vi "Parse Uplink.vi"(8 "error in (no error)":errorcluster, 10 "Uplink":u8[][](array[numeric]) format="%02x") -> (0 "error out":errorcluster, 1 "Data":string, 2 "Response Code":string, 3 "Response Token":string, 4 "tChecksum Valid":bool, 5 "CP_DATA":u8[](array[numeric]), 6 "bChecksum Valid":bool)   [LabVIEW 2020]
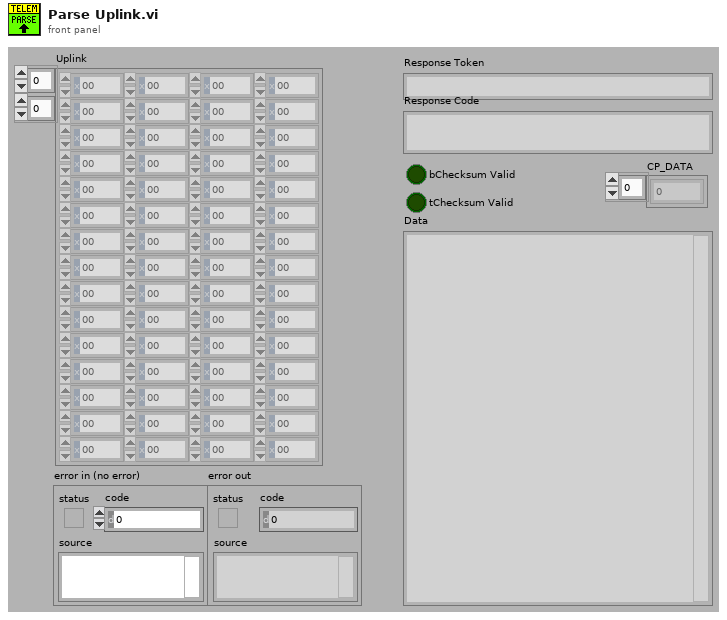
[diagram p1: front panel]
types:
  T1 = cluster{"FirstBlockFlag":u8, "respToken":u8, "cmdToken":u16, "cmdData":u8[], "b1ChkSum":u8, "tChkSum":u8, "tChkSumCalc":u8, "b1ChkSumCalc":u8}
  T2 = cluster{"Boolean array[0]":bool, "Boolean array[1]":bool, "Boolean array[2]":bool, "Boolean array[3]":bool, "Boolean array[4]":bool, "Boolean array[5]":bool, "Boolean array[6]":bool, "Boolean array[7]":bool}
  T3 = cluster{"Boolean array[0]":bool, "Boolean array[1]":bool, "Boolean array[2]":bool, "Boolean array[3]":bool, "Boolean array[4]":bool, "Boolean array[5]":bool, "Boolean array[6]":bool, "Boolean array[7]":bool, "Boolean array[8]":bool, "Boolean array[9]":bool, "Boolean array[10]":bool, "Boolean array[11]":bool, "Boolean array[12]":bool, "Boolean array[13]":bool, "Boolean array[14]":bool, "Boolean array[15]":bool}
  T4 = cluster{"DATA[0]":u8, "DATA[1]":u8, "DATA[2]":u8, "DATA[3]":u8, "DATA[4]":u8, "DATA[5]":u8, "DATA[6]":u8, "DATA[7]":u8}
  T5 = cluster{"[0]":string, "[1]":string, "[2]":string, "[3]":string, "[4]":string, "[5]":string, "[6]":string, "[7]":string, "[8]":string, "[9]":string}
  T6 = cluster{"DATA[0]":u8, "DATA[1]":u8, "DATA[2]":u8, "DATA[3]":u8, "DATA[4]":u8, "DATA[5]":u8, "DATA[6]":u8, "DATA[7]":u8, "DATA[8]":u8, "DATA[9]":u8, "DATA[10]":u8, "DATA[11]":u8, "DATA[12]":u8, "DATA[13]":u8, "DATA[14]":u8, "DATA[15]":u8}
  T7 = cluster{"[0]":u8, "[1]":u8, "[2]":u8, "[3]":u8, "[4]":u8, "[5]":u8, "[6]":u8, "[7]":u8, "[8]":u8, "[9]":u8, "[10]":u8, "[11]":u8, "[12]":u8, "[13]":u8, "[14]":u8, "[15]":u8, "[16]":u8, "[17]":u8, "[18]":u8, "[19]":u8, "[20]":u8, "[21]":u8, "[22]":u8, "[23]":u8, "[24]":u8, "[25]":u8, "[26]":u8, "[27]":u8, "[28]":u8, "[29]":u8, "[30]":u8, "[31]":u8, "[32]":u8, "[33]":u8, "[34]":u8, "[35]":u8, "[36]":u8, "[37]":u8, "[38]":u8, "[39]":u8, "[40]":u8, "[41]":u8, "[42]":u8, "[43]":u8, "[44]":u8, "[45]":u8, "[46]":u8, "[47]":u8, "[48]":u8, "[49]":u8, "[50]":u8, "[51]":u8, "[52]":u8, "[53]":u8}
  T8 = cluster{"DATA[0]":u8, "DATA[1]":u8, "DATA[2]":u8, "DATA[3]":u8, "DATA[4]":u8, "DATA[5]":u8, "DATA[6]":u8, "DATA[7]":u8, "DATA[8]":u8, "DATA[9]":u8, "DATA[10]":u8, "DATA[11]":u8, "DATA[12]":u8, "DATA[13]":u8, "DATA[14]":u8, "DATA[15]":u8, "DATA[16]":u8, "DATA[17]":u8, "DATA[18]":u8, "DATA[19]":u8, "DATA[20]":u8, "DATA[21]":u8, "DATA[22]":u8, "DATA[23]":u8, "DATA[24]":u8, "DATA[25]":u8, "DATA[26]":u8, "DATA[27]":u8, "DATA[28]":u8, "DATA[29]":u8, "DATA[30]":u8, "DATA[31]":u8, "DATA[32]":u8, "DATA[33]":u8, "DATA[34]":u8, "DATA[35]":u8, "DATA[36]":u8, "DATA[37]":u8, "DATA[38]":u8, "DATA[39]":u8, "DATA[40]":u8, "DATA[41]":u8, "DATA[42]":u8, "DATA[43]":u8, "DATA[44]":u8, "DATA[45]":u8, "DATA[46]":u8}
  T9 = cluster{"DATA[0]":u8, "DATA[1]":u8, "DATA[2]":u8, "DATA[3]":u8, "DATA[4]":u8, "DATA[5]":u8, "DATA[6]":u8, "DATA[7]":u8, "DATA[8]":u8, "DATA[9]":u8, "DATA[10]":u8, "DATA[11]":u8, "DATA[12]":u8, "DATA[13]":u8, "DATA[14]":u8, "DATA[15]":u8, "DATA[16]":u8, "DATA[17]":u8, "DATA[18]":u8, "DATA[19]":u8, "DATA[20]":u8, "DATA[21]":u8, "DATA[22]":u8, "DATA[23]":u8}
  T10 = cluster{"Boolean array[0]":bool, "Boolean array[1]":bool, "Boolean array[2]":bool, "Boolean array[3]":bool, "Boolean array[4]":bool, "Boolean array[5]":bool, "Boolean array[6]":bool, "Boolean array[7]":bool, "Boolean array[8]":bool}
  T11 = cluster{"[0]":u8, "[1]":u8, "[2]":u8, "[3]":u8, "[4]":u8, "[5]":u8, "[6]":u8, "[7]":u8, "[8]":u8, "[9]":u8}
  T12 = cluster{"DATA[0]":u8, "DATA[1]":u8, "DATA[2]":u8, "DATA[3]":u8, "DATA[4]":u8, "DATA[5]":u8, "DATA[6]":u8, "DATA[7]":u8, "DATA[8]":u8}
  T13 = cluster{"[0]":u8, "[1]":u8, "[2]":u8, "[3]":u8, "[4]":u8, "[5]":u8, "[6]":u8, "[7]":u8, "[8]":u8, "[9]":u8, "[10]":u8, "[11]":u8, "[12]":u8, "[13]":u8, "[14]":u8, "[15]":u8, "[16]":u8, "[17]":u8, "[18]":u8, "[19]":u8, "[20]":u8, "[21]":u8, "[22]":u8, "[23]":u8, "[24]":u8, "[25]":u8, "[26]":u8, "[27]":u8, "[28]":u8, "[29]":u8, "[30]":u8, "[31]":u8, "[32]":u8, "[33]":u8, "[34]":u8, "[35]":u8, "[36]":u8, "[37]":u8}
  T14 = cluster{"[0]":u8, "[1]":u8, "[2]":u8, "[3]":u8, "[4]":u8, "[5]":u8}
  T15 = cluster{"DATA[0]":u8, "DATA[1]":u8, "DATA[2]":u8, "DATA[3]":u8, "DATA[4]":u8, "DATA[5]":u8}
  T16 = cluster{"DATA[0]":u8, "DATA[1]":u8, "DATA[2]":u8, "DATA[3]":u8, "DATA[4]":u8, "DATA[5]":u8, "DATA[6]":u8, "DATA[7]":u8, "DATA[8]":u8, "DATA[9]":u8, "DATA[10]":u8, "DATA[11]":u8, "DATA[12]":u8, "DATA[13]":u8, "DATA[14]":u8, "DATA[15]":u8, "DATA[16]":u8}
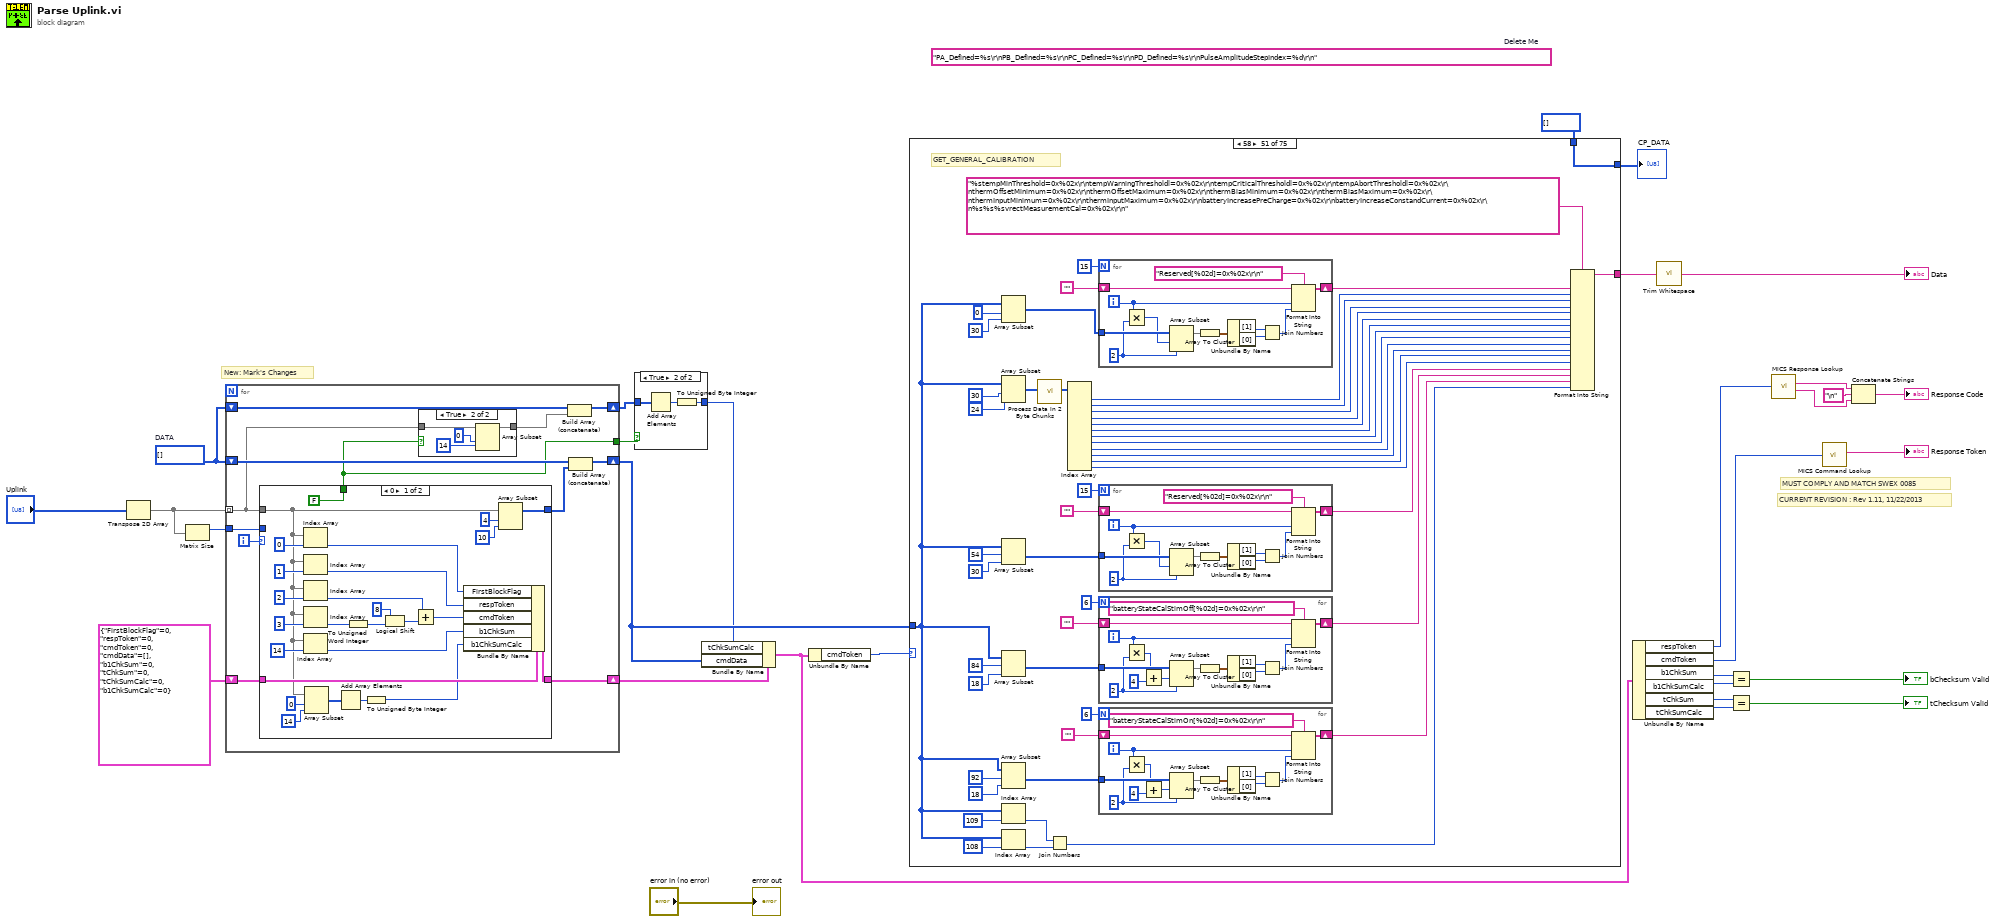
[diagram p0: block diagram]
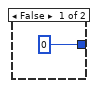
[diagram p2: hidden frame]
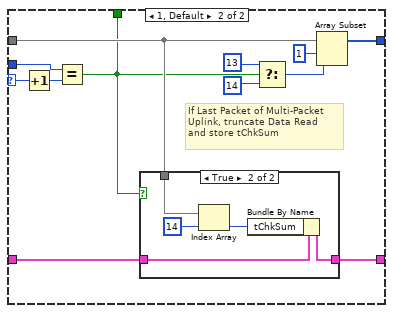
[diagram p4: hidden frame]
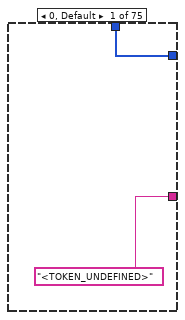
[diagram p6: hidden frame]
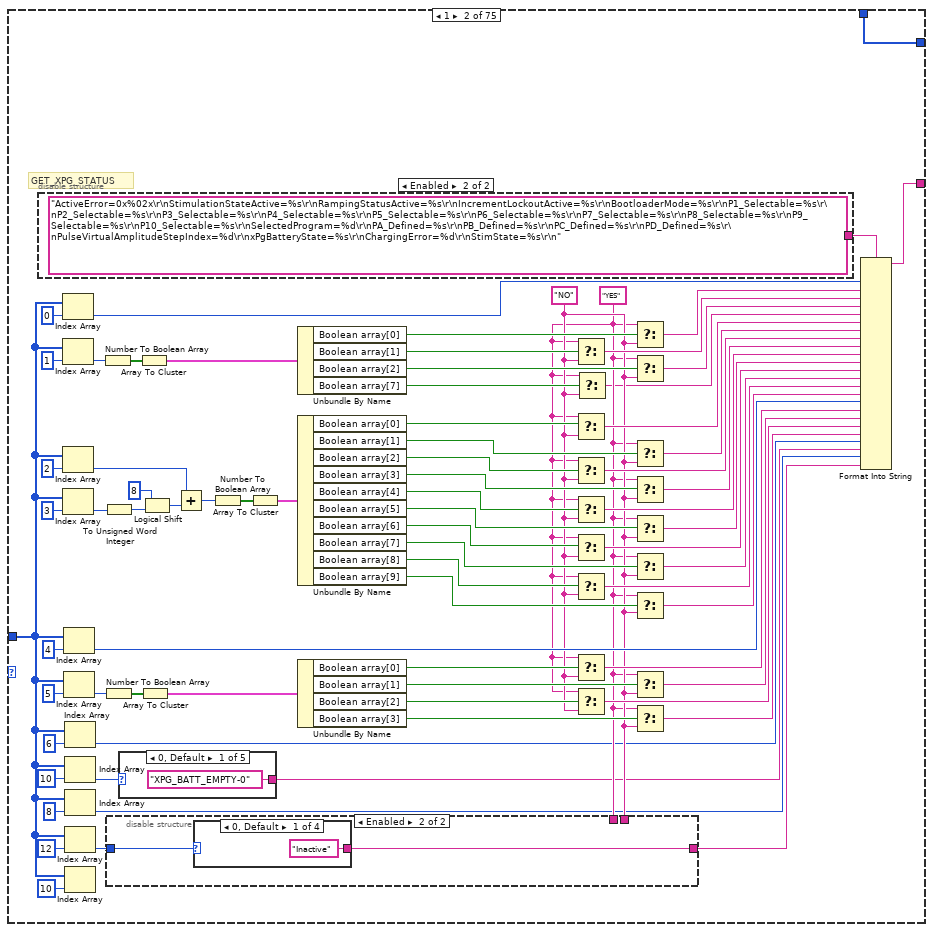
[diagram p7: hidden frame]
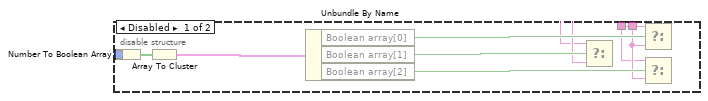
[diagram p8: hidden frame]
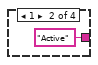
[diagram p9: hidden frame]
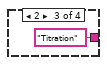
[diagram p10: hidden frame]
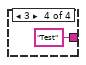
[diagram p11: hidden frame]
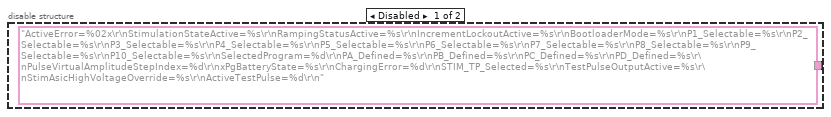
[diagram p12: hidden frame]
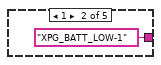
[diagram p13: hidden frame]
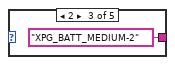
[diagram p14: hidden frame]
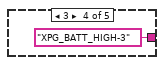
[diagram p15: hidden frame]
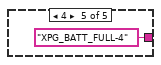
[diagram p16: hidden frame]
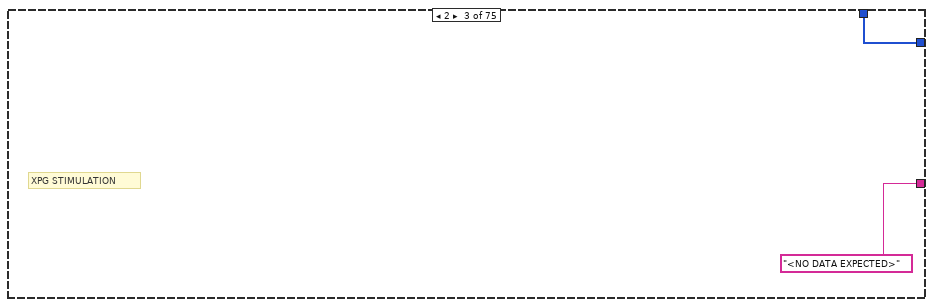
[diagram p17: hidden frame]
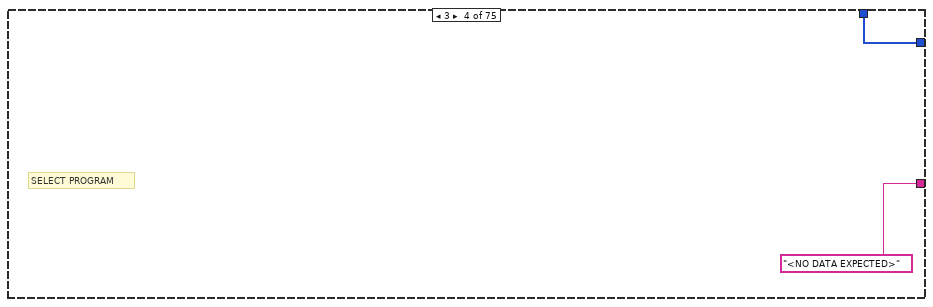
[diagram p18: hidden frame]
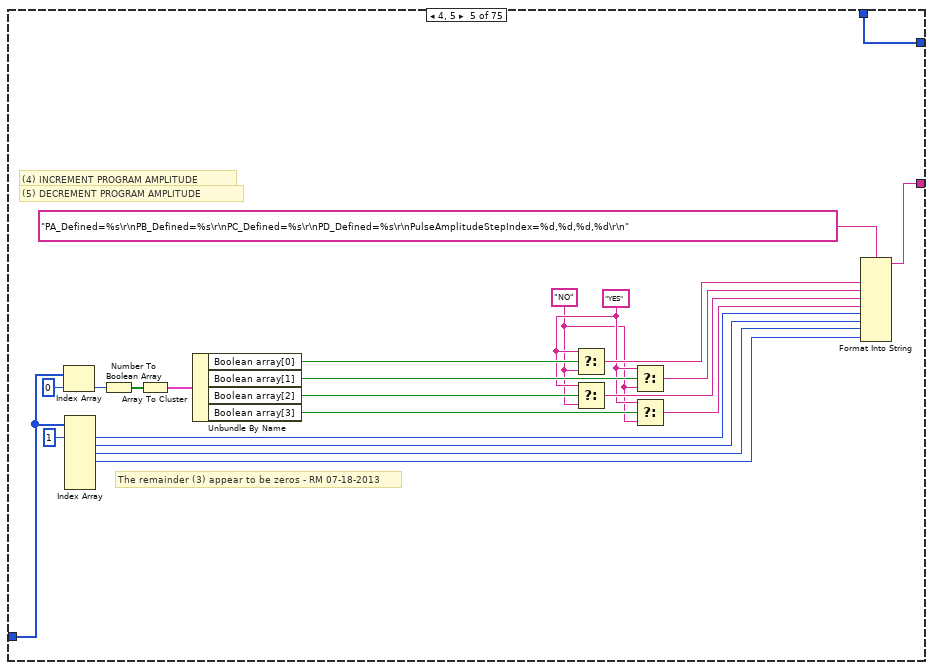
[diagram p19: hidden frame]
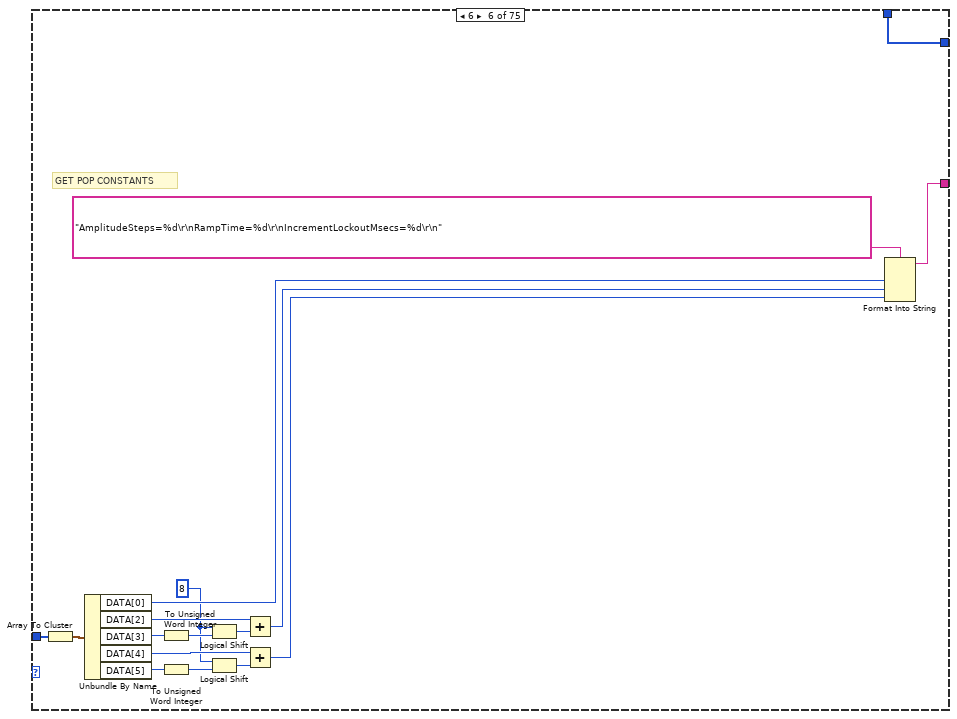
[diagram p20: hidden frame]
diagram:
  w14 = u8[] []  # DATA
  (unwired) "PA_Defined=%s\r\nPB_Defined=%s\r\nPC_Defined=%s\r\nPD_Defined=%s\r\nPulseAmplitudeStepIndex=%d\r\n"  # Delete Me
  # "CURRENT REVISION : Rev 1.11, 11/22/2013"
  # "MUST COMPLY AND MATCH SWEX 0085"
  # "New: Mark's Changes"
  n1 = Transpose 2D Array(2D array="Uplink") -> (transposed array=w13:u8[][])
  n2 = Matrix Size(0:w13) -> (1:w11:i32)  [unwired: 1 out]
  n3 = for {
    tunnel: w13 -> [w33] mode=indexing
    shift-right: [w37] -> w30
    shift-left: w14 -> [w38]
    shift-right: [w40] -> w12
    shift-left: T1 {"FirstBlockFlag"=0, "respToken"=0, "cmdToken"=0, "cmdData"=[], "b1ChkSum"=0, "tChkSum"=0, "tChkSumCalc"=0, "b1ChkSumCalc"=0} -> [w41]
    tunnel: w11 -> [w39]
    shift-right: [w34] -> w15
    shift-left: w14 -> [w35]
    tunnel: [w31] -> w16
    i -> [w42]
    n4 = case shown="0" w42 {
      selector: w42 -> [_ w85]
      tunnel: w33 -> [w51 w75]
      tunnel: [w71 w81] -> w36
      tunnel: w41 -> [w65 w76]
      tunnel: [w64 w77] -> w40
      tunnel: w39 -> [_ w83]
      tunnel: [FALSE w74] -> w31
      frame 0 {
        n5 = Index Array(array=w51, index=0) -> (element=w63:u8)
        n6 = Index Array(array=w51, index=1) -> (element=w60:u8)
        n7 = Index Array(array=w51, index=2) -> (element=w55:u8)
        n8 = Index Array(array=w51, index=3) -> (element=w59:u8)
        n9 = Index Array(array=w51, index=14) -> (element=w62:u8)
        n10 = Array Subset(array=w51, index=0, length=14) -> (w48:u8[])
        n11 = Add Array Elements(numeric array=w48) -> (sum=w50:u8)
        n12 = To Unsigned Word Integer(number=w59) -> (unsigned 16bit integer=w61:u16)
        n13 = To Unsigned Byte Integer(number=w50) -> (unsigned 8bit integer=w49:u8)
        n14 = Logical Shift(y=i8 8, x=w61) -> (x << y=w57:u16)
        n15 = Add(x=w55, y=w57) -> (x+y=w56:u16)
        n16 = Bundle By Name(cluster=w65, "FirstBlockFlag"=w63, "respToken"=w60, "cmdToken"=w56, "b1ChkSum"=w62, "b1ChkSumCalc"=w49) -> (w64:T1)
        n17 = Array Subset(array=w51, index=4, length=10) -> (w71:u8[])
      }
      frame 1, Default {
        # "If Last Packet of Multi-Packet\nUplink, truncate Data Read\nand store tChkSum"
        n18 = Increment(x=w85) -> (x+1=w84:i32)
        n19 = Equal?(x=w83, y=w84) -> (x = y?=w74:bool)
        n20 = case shown="True" w74 {
          tunnel: [w86 w90] -> w77
          tunnel: w76 -> [w86 w91]
          tunnel: w75 -> [_ w88]
          frame False {
          }
          frame True {
            n21 = Index Array(array=w88, index=14) -> (element=w89:u8)
            n22 = Bundle By Name(cluster=w91, "tChkSum"=w89) -> (w90:T1)
          }
        }
        n23 = Select(t=13 ("length"), s=w74, f=14 ("length")) -> (s? t:f=w80:i32)
        n24 = Array Subset(array=w75, index=1, length=w80) -> (w81:u8[])
      }
    }
    n25 = case shown="True" w31 {
      tunnel: w33 -> [w43 w46]
      tunnel: [w43 w45] -> w32
      frame False {
      }
      frame True {
        n26 = Array Subset(array=w46, index=0, length=14) -> (w45:u8[])
      }
    }
    n27 = Build Array (concatenate)(w35, w32) -> (w34:u8[])
    n28 = Build Array (concatenate)(w38, w36) -> (w37:u8[])
  }
  n29 = case shown="True" w16 {
    tunnel: w15 -> [_ w93]
    tunnel: [u16 0 ("CRC16r") w94] -> w17
    frame False {
    }
    frame True {
      n30 = Add Array Elements(numeric array=w93) -> (sum=w95:u8)
      n31 = To Unsigned Byte Integer(number=w95) -> (unsigned 8bit integer=w94:u8)
    }
  }
  n32 = Bundle By Name(cluster=w12, "tChkSumCalc"=w17, "cmdData"=w30) -> (w21:T1)
  n33 = Unbundle By Name(w21) -> ("cmdToken"=w18:u16)
  n34 = case shown="58" w18 {
    tunnel: w30 -> [_ w108 _ _ w209 w228 w238 w321 w368 w374 w380 w397 _ w418 w424 w430 _ w438 w444 _ w461 w488 _ _ w499 _ w638 _ w665 _ w817 _ w828 _ w888 _ w937 _ w971 _ _ w1002 w1037 w1060 w1081 _ w1091 _ w1103 w1109 w1131 _ w1219 _ w1269 _ w1276 _ w1338 _ w1396 _ w1403 _ _ _ w1424 _ _ _ _ w1447 _ w1505 _]
    tunnel: ["<TOKEN_UNDEFINED>" w170 "<NO DATA EXPECTED>" "<NO DATA EXPECTED>" w219 w235 w297 w354 w369 w375 w381 w411 "<NO DATA EXPECTED>" w419 w425 w431 "<NO DATA EXPECTED>" w439 w445 "<NO DATA EXPECTED>" w462 w475 "<NO DATA EXPECTED>" "<NO DATA EXPECTED>" w538 "<NO DATA EXPECTED>" w641 "<NO DATA EXPECTED>" w730 "<NO DATA EXPECTED>" w821 "<NO DATA EXPECTED>" w833 "<NO DATA EXPECTED>" w893 "<NO DATA EXPECTED>" w940 "<NO DATA EXPECTED>" w973 "<NO DATA EXPECTED>" "<NO DATA EXPECTED>" ("format string") w1003 w1039 w1062 w1083 "<NO DATA EXPECTED>" w1095 "<NO DATA EXPECTED>" w1105 w1113 w1162 "<NO DATA EXPECTED>" w1220 "<NO DATA EXPECTED>" w1270 "<NO DATA EXPECTED>" w1284 "<NO DATA EXPECTED>" w1345 "<NO DATA EXPECTED>" w1397 "<NO DATA EXPECTED>" w1411 _ _ "<NO DATA EXPECTED>" w1432 "<NO DATA EXPECTED>" _ _ _ w1448 "<NO DATA EXPECTED>" w1507 "<TOKEN_UNDEFINED (0x7FAA)>"] -> w29
    tunnel: [w96 w98 w193 w195 w197 w220 w237 w307 w365 w371 w377 w383 w413 w415 w421 w427 w433 w435 w441 w447 w449 w474 w493 w495 w497 w634 w636 w660 w662 w740 w742 w823 w825 w873 w875 w933 w935 w960 w969 w980 w982 w984 w1035 w1051 w1080 w1085 w1087 w1097 w1099 w1107 w1115 w1216 w1218 w1257 w1259 w1272 w1274 w1334 w1336 w1386 w1388 w1399 w1401 w1412 w1413 w1414 w1416 w1442 w1443 w1444 w1445 w1446 w1497 w1499 w1510] -> w2
    tunnel: u8[] [] -> [w96 w98 w193 w195 w197 w220 w237 w307 w365 w371 w377 w383 w413 w415 w421 w427 w433 w435 w441 w447 w449 w474 w493 w495 w497 w634 w636 w660 w662 w740 w742 w823 w825 w873 w875 w933 w935 w960 _ w980 w982 w984 w1035 w1051 w1080 w1085 w1087 w1097 w1099 w1107 w1115 w1216 w1218 w1257 w1259 w1272 w1274 w1334 w1336 w1386 w1388 w1399 w1401 w1412 w1413 w1414 _ w1442 w1443 w1444 w1445 w1446 w1497 w1499 w1510]
    frame 0, Default {
    }
    frame 1 {
      w106 = "NO"
      w105 = "YES"
      # "GET_XPG_STATUS"
      n35 = disable-structure shown="Enabled" {
        disable-tunnel: [_ "ActiveError=0x%02x\r\nStimulationStateActive=%s\r\nRampingStatusActive=%s\r\nIncrementLockoutActive=%s\r\nBootloaderMode=%s\r\nP1_Selectable=%s\r\nP2_Selectable=%s\r\nP3_Selectable=%s\r\nP4_Selectable=%s\r\nP5_Selectable=%s\r\nP6_Selectable=%s\r\nP7_Selectable=%s\r\nP8_Selectable=%s\r\nP9_Selectable=%s\r\nP10_Selectable=%s\r\nSelectedProgram=%d\r\nPA_Defined=%s\r\nPB_Defined=%s\r\nPC_Defined=%s\r\nPD_Defined=%s\r\nPulseVirtualAmplitudeStepIndex=%d\r\nxPgBatteryState=%s\r\nChargingError=%d\r\nStimState=%s\r\n" ("format string")] -> w99
        frame Disabled {
          (unwired) "ActiveError=%02x\r\nStimulationStateActive=%s\r\nRampingStatusActive=%s\r\nIncrementLockoutActive=%s\r\nBootloaderMode=%s\r\nP1_Selectable=%s\r\nP2_Selectable=%s\r\nP3_Selectable=%s\r\nP4_Selectable=%s\r\nP5_Selectable=%s\r\nP6_Selectable=%s\r\nP7_Selectable=%s\r\nP8_Selectable=%s\r\nP9_Selectable=%s\r\nP10_Selectable=%s\r\nSelectedProgram=%d\r\nPA_Defined=%s\r\nPB_Defined=%s\r\nPC_Defined=%s\r\nPD_Defined=%s\r\nPulseVirtualAmplitudeStepIndex=%d\r\nxPgBatteryState=%s\r\nChargingError=%d\r\nSTIM_TP_Selected=%s\r\nTestPulseOutputActive=%s\r\nStimAsicHighVoltageOverride=%s\r\nActiveTestPulse=%d\r\n" ("format string")
        }
        frame Enabled {
        }
      }
      n36 = Index Array(array=w108, index=0) -> (element=w171:u8)
      n37 = Index Array(array=w108, index=1) -> (element=w155:u8)
      n38 = Index Array(array=w108, index=2) -> (element=w143:u8)
      n39 = Index Array(array=w108, index=3) -> (element=w144:u8)
      n40 = Index Array(array=w108, index=4) -> (element=w128:u8)
      n41 = Index Array(array=w108, index=5) -> (element=w126:u8)
      n42 = Index Array(array=w108, index=6) -> (element=w103:u8)
      n43 = Index Array(array=w108, index=10) -> (element=w113:u8)
      n44 = Index Array(array=w108, index=8) -> (element=w101:u8)
      n45 = Index Array(array=w108, index=12) -> (element=w110:u8)
      n46 = Index Array(array=w108, index=10) -> ()  [unwired: 1 out]
      n47 = Number To Boolean Array(number=w155) -> (Boolean array=w154:bool[])
      n48 = To Unsigned Word Integer(number=w144) -> (unsigned 16bit integer=w147:u16)
      n49 = Number To Boolean Array(number=w126) -> (Boolean array=w125:bool[])
      n50 = disable-structure shown="Enabled" {
        disable-tunnel: w110 -> [w180 w182]
        disable-tunnel: w106 -> [w174 _]
        disable-tunnel: w105 -> [w173 _]
        disable-tunnel: [_ w181] -> w100
        frame Disabled {
          n51 = Number To Boolean Array(number=w180) -> (Boolean array=w179:bool[])
          n52 = Array To Cluster(array=w179) -> (cluster=w178:T2)
          n53 = Unbundle By Name(w178) -> ("Boolean array[0]"=w177:bool, "Boolean array[1]"=w176:bool, "Boolean array[2]"=w175:bool)
          n54 = Select(t=w173, s=w176, f=w174) -> ()  [unwired: 1 out]
          n55 = Select(t=w173, s=w177, f=w174) -> ()  [unwired: 1 out]
          n56 = Select(t=w173, s=w175, f=w174) -> ()  [unwired: 1 out]
        }
        frame Enabled {
          n57 = case shown="0, Default" w182 {
            tunnel: ["Inactive" "Active" "Titration" "Test"] -> w181
            frame 0, Default {
            }
            frame 1 {
            }
            frame 2 {
            }
            frame 3 {
            }
          }
        }
      }
      n58 = case shown="0, Default" w113 {
        tunnel: ["XPG_BATT_EMPTY-0" "XPG_BATT_LOW-1" "XPG_BATT_MEDIUM-2" "XPG_BATT_HIGH-3" "XPG_BATT_FULL-4"] -> w102
        frame 0, Default {
        }
        frame 1 {
        }
        frame 2 {
        }
        frame 3 {
        }
        frame 4 {
        }
      }
      n59 = Array To Cluster(array=w154) -> (cluster=w153:T2)
      n60 = Array To Cluster(array=w125) -> (cluster=w124:T2)
      n61 = Logical Shift(y=i8 8, x=w147) -> (x << y=w145:u16)
      n62 = Add(x=w143, y=w145) -> (x+y=w141:u16)
      n63 = Number To Boolean Array(number=w141) -> (Boolean array=w142:bool[])
      n64 = Array To Cluster(array=w142) -> (cluster=w140:T3)
      n65 = Unbundle By Name(w153) -> ("Boolean array[0]"=w152:bool, "Boolean array[1]"=w151:bool, "Boolean array[2]"=w150:bool, "Boolean array[7]"=w107:bool)
      n66 = Unbundle By Name(w140) -> ("Boolean array[0]"=w139:bool, "Boolean array[1]"=w138:bool, "Boolean array[2]"=w137:bool, "Boolean array[3]"=w136:bool, "Boolean array[4]"=w135:bool, "Boolean array[5]"=w134:bool, "Boolean array[6]"=w133:bool, "Boolean array[7]"=w132:bool, "Boolean array[8]"=w131:bool, "Boolean array[9]"=w130:bool)
      n67 = Unbundle By Name(w124) -> ("Boolean array[0]"=w123:bool, "Boolean array[1]"=w122:bool, "Boolean array[2]"=w121:bool, "Boolean array[3]"=w120:bool)
      n68 = Select(t=w105, s=w151, f=w106) -> (s? t:f=w168:string)
      n69 = Select(t=w105, s=w139, f=w106) -> (s? t:f=w166:string)
      n70 = Select(t=w105, s=w137, f=w106) -> (s? t:f=w164:string)
      n71 = Select(t=w105, s=w135, f=w106) -> (s? t:f=w162:string)
      n72 = Select(t=w105, s=w133, f=w106) -> (s? t:f=w160:string)
      n73 = Select(t=w105, s=w131, f=w106) -> (s? t:f=w158:string)
      n74 = Select(t=w105, s=w123, f=w106) -> (s? t:f=w119:string)
      n75 = Select(t=w105, s=w121, f=w106) -> (s? t:f=w117:string)
      n76 = Select(t=w105, s=w107, f=w106) -> (s? t:f=w104:string)
      n77 = Select(t=w105, s=w152, f=w106) -> (s? t:f=w169:string)
      n78 = Select(t=w105, s=w150, f=w106) -> (s? t:f=w167:string)
      n79 = Select(t=w105, s=w138, f=w106) -> (s? t:f=w165:string)
      n80 = Select(t=w105, s=w136, f=w106) -> (s? t:f=w163:string)
      n81 = Select(t=w105, s=w134, f=w106) -> (s? t:f=w161:string)
      n82 = Select(t=w105, s=w132, f=w106) -> (s? t:f=w159:string)
      n83 = Select(t=w105, s=w130, f=w106) -> (s? t:f=w157:string)
      n84 = Select(t=w105, s=w122, f=w106) -> (s? t:f=w118:string)
      n85 = Select(t=w105, s=w120, f=w106) -> (s? t:f=w116:string)
      n86 = Format Into String(format string=w99, w171, w169, w168, w167, w104, w166, w165, w164, w163, w162, w161, w160, w159, w158, w157, w128, w119, w118, w117, w116, w103, w102, w101, w100) -> (resulting string=w170:string)  [unwired: 2 in, 1 out]
    }
    frame 2 {
      # "XPG STIMULATION"
    }
    frame 3 {
      # "SELECT PROGRAM"
    }
    frame 4, 5 {
      w202 = "NO"
      w203 = "YES"
      # "(5) DECREMENT PROGRAM AMPLITUDE"
      # "(4) INCREMENT PROGRAM AMPLITUDE"
      # "The remainder (3) appear to be zeros - RM 07-18-2013"
      n87 = Index Array(array=w209, index=0) -> (element=w217:u8)
      n88 = Index Array(array=w209, index #1=1 ("index")) -> (element #1=w204:u8, element #2=w200:u8, element #3=w199:u8, element #4=w198:u8)  [unwired: 6 in, 3 out]
      n89 = Number To Boolean Array(number=w217) -> (Boolean array=w216:bool[])
      n90 = Array To Cluster(array=w216) -> (cluster=w215:T2)
      n91 = Unbundle By Name(w215) -> ("Boolean array[0]"=w214:bool, "Boolean array[1]"=w213:bool, "Boolean array[2]"=w212:bool, "Boolean array[3]"=w211:bool)
      n92 = Select(t=w203, s=w214, f=w202) -> (s? t:f=w208:string)
      n93 = Select(t=w203, s=w212, f=w202) -> (s? t:f=w206:string)
      n94 = Select(t=w203, s=w213, f=w202) -> (s? t:f=w207:string)
      n95 = Select(t=w203, s=w211, f=w202) -> (s? t:f=w205:string)
      n96 = Format Into String(format string="PA_Defined=%s\r\nPB_Defined=%s\r\nPC_Defined=%s\r\nPD_Defined=%s\r\nPulseAmplitudeStepIndex=%d,%d,%d,%d\r\n", w208, w207, w206, w205, w204, w200, w199, w198) -> (resulting string=w219:string)  [unwired: 2 in, 1 out]
    }
    frame 6 {
      w221 = i8 8 ("y")
      # "GET POP CONSTANTS"
      n97 = Array To Cluster(array=w228) -> (cluster=w227:T4)
      n98 = Unbundle By Name(w227) -> ("DATA[0]"=w226:u8, "DATA[2]"=w225:u8, "DATA[3]"=w224:u8, "DATA[4]"=w223:u8, "DATA[5]"=w222:u8)
      n99 = To Unsigned Word Integer(number=w224) -> (unsigned 16bit integer=w234:u16)
      n100 = To Unsigned Word Integer(number=w222) -> (unsigned 16bit integer=w232:u16)
      n101 = Logical Shift(y=w221, x=w234) -> (x << y=w233:u16)
      n102 = Logical Shift(y=w221, x=w232) -> (x << y=w231:u16)
      n103 = Add(x=w225, y=w233) -> (x+y=w230:u16)
      n104 = Add(x=w223, y=w231) -> (x+y=w229:u16)
      n105 = Format Into String(format string="AmplitudeSteps=%d\r\nRampTime=%d\r\nIncrementLockoutMsecs=%d\r\n", w226, w230, w229) -> (resulting string=w235:string)  [unwired: 2 in, 1 out]
    }
    frame 7 {
      w240 = "NO"
      w278 = "YES"
      # "Convert MS DateTime\nto LV DateTime"
      # "GET PPC CONSTANTS"
      n106 = Array Subset(array=w238, index=0, length=30) -> (w294:u8[])
      n107 = Index Array(array=w238, index=30) -> (element=w286:u8)
      n108 = Index Array(array=w238, index=31) -> (element=w287:u8)
      n109 = Index Array(array=w238, index=32) -> (element=w283:u8)
      n110 = Index Array(array=w238, index=33) -> (element=w281:u8)
      n111 = Index Array(array=w238, index=34) -> (element=w265:u8)
      n112 = Index Array(array=w238, index=35) -> (element=w266:u8)
      n113 = Index Array(array=w238, index=36) -> (element=w257:u8)
      n114 = Index Array(array=w238, index=37) -> (element=w258:u8)
      n115 = Array Subset(array=w238, index=38, length=8) -> (w253:u8[])
      n116 = Index Array(array=w238, index=46) -> (element=w243:u8)
      n117 = Number To Boolean Array(number=w281) -> (Boolean array=w280:bool[])
      n118 = To Unsigned Word Integer(number=w287) -> (unsigned 16bit integer=w290:u16)
      n119 = To Unsigned Word Integer(number=w266) -> (unsigned 16bit integer=w269:u16)
      n120 = To Unsigned Word Integer(number=w258) -> (unsigned 16bit integer=w261:u16)
      n121 = Byte Array To String(unsigned byte array=w294) -> (string=w293:string)
      n122 = Array To Cluster(array=w280) -> (cluster=w279:T2)
      n123 = Logical Shift(y=i8 8, x=w290) -> (x << y=w288:u16)
      n124 = Logical Shift(y=i8 8, x=w269) -> (x << y=w267:u16)
      n125 = Logical Shift(y=i8 8, x=w261) -> (x << y=w259:u16)
      n126 = for {
        tunnel: w253 -> [w306] mode=indexing
        shift-right: [w300] -> w248
        shift-left: u64 0 ("y") -> [w301]
        tunnel: i8 8 ("y") -> [w304]
        i -> [w305]
        n127 = To Unsigned Quad Integer(1:w306) -> (0:w299:u64)
        n128 = Multiply(x=w304, y=w305) -> (x*y=w303:i32)
        n129 = Logical Shift(y=w303, x=w299) -> (x << y=w302:u64)
        n130 = Add(x=w301, y=w302) -> (x+y=w300:u64)
      }
      n131 = Add(x=w286, y=w288) -> (x+y=w285:u16)
      n132 = Unbundle By Name(w279) -> ("Boolean array[0]"=w276:bool, "Boolean array[1]"=w277:bool, "Boolean array[2]"=w275:bool)
      n133 = Add(x=w265, y=w267) -> (x+y=w264:u16)
      n134 = Add(x=w257, y=w259) -> (x+y=w256:u16)
      n135 = Select(t=w278, s=w276, f=w240) -> (s? t:f=w274:string)
      n136 = Select(t=w278, s=w275, f=w240) -> (s? t:f=w272:string)
      n137 = Multiply(x=u64 1904 ("y"), y=u64 31556926) -> (x*y=w246:u64)
      n138 = Quotient & Remainder(x=w248, y=u64 10000000) -> (floor(x/y)=w239:u64)  [unwired: 1 out]
      n139 = Select(t=w278, s=w277, f=w240) -> (s? t:f=w273:string)
      n140 = Subtract(x=w239, y=w246) -> (x-y=w242:u64)
      n141 = Format Date/Time String(seconds (now)=w242, UTC format=FALSE) -> (date/time string=w241:string)  [unwired: 1 in]
      n142 = Format Into String(format string="PPCText=%s\r\nPulseWidthStep=%d\r\nAmplitudeSteps=%d\r\nAllowIndividualPulseAmplitudeModification=%s\r\nAllowIndividualPulseWidthModification=%s\r\nAllowProgramFrequencyModification=%s\r\nRampTime=%d\r\nIncrementalLockoutMsecs=%d\r\nImplantDateTime=%s\r\nReplacementIntervalMonths=%d\r\n", w293, w285, w283, w274, w273, w272, w264, w256, w241, w243) -> (resulting string=w297:string)  [unwired: 2 in, 1 out]
    }
    frame 8 {
      w333 = "NO"
      w332 = "YES"
      # "GET_PROGRAM_NAMES"
      n143 = Index Array(array=w321, index=0) -> (element=w347:u8)
      n144 = Index Array(array=w321, index=1) -> (element=w348:u8)
      n145 = To Unsigned Word Integer(number=w348) -> (unsigned 16bit integer=w351:u16)
      n146 = Logical Shift(y=i8 8, x=w351) -> (x << y=w349:u16)
      n147 = Add(x=w347, y=w349) -> (x+y=w345:u16)
      n148 = for {
        N: 10 -> [_]
        tunnel: w321 -> [w364]
        tunnel: [w356] -> w320 mode=indexing
        i -> [w362]
        n149 = Multiply(x=16, y=w362) -> (x*y=w360:i32)
        n150 = Add(x=2, y=w360) -> (x+y=w358:i32)
        n151 = Array Subset(array=w364, index=w358, length=10) -> (w357:u8[])
        n152 = Byte Array To String(unsigned byte array=w357) -> (string=w356:string)
      }
      n153 = Number To Boolean Array(number=w345) -> (Boolean array=w346:bool[])
      n154 = Array To Cluster(array=w346) -> (cluster=w344:T3)
      n155 = Unbundle By Name(w344) -> ("Boolean array[0]"=w343:bool, "Boolean array[1]"=w342:bool, "Boolean array[2]"=w341:bool, "Boolean array[3]"=w340:bool, "Boolean array[4]"=w339:bool, "Boolean array[5]"=w338:bool, "Boolean array[6]"=w337:bool, "Boolean array[7]"=w336:bool, "Boolean array[8]"=w335:bool, "Boolean array[9]"=w334:bool)
      n156 = Array To Cluster(array=w320) -> (cluster=w319:T5)
      n157 = Unbundle(w319) -> ("[0]"=w317:string, "[1]"=w316:string, "[2]"=w315:string, "[3]"=w314:string, "[4]"=w313:string, "[5]"=w312:string, "[6]"=w311:string, "[7]"=w310:string, "[8]"=w309:string, "[9]"=w308:string)
      n158 = Select(t=w332, s=w343, f=w333) -> (s? t:f=w331:string)
      n159 = Select(t=w332, s=w341, f=w333) -> (s? t:f=w329:string)
      n160 = Select(t=w332, s=w339, f=w333) -> (s? t:f=w327:string)
      n161 = Select(t=w332, s=w337, f=w333) -> (s? t:f=w325:string)
      n162 = Select(t=w332, s=w335, f=w333) -> (s? t:f=w323:string)
      n163 = Select(t=w332, s=w342, f=w333) -> (s? t:f=w330:string)
      n164 = Select(t=w332, s=w340, f=w333) -> (s? t:f=w328:string)
      n165 = Select(t=w332, s=w338, f=w333) -> (s? t:f=w326:string)
      n166 = Select(t=w332, s=w336, f=w333) -> (s? t:f=w324:string)
      n167 = Select(t=w332, s=w334, f=w333) -> (s? t:f=w322:string)
      n168 = Format Into String(format string="P1_Selectable=%s\r\nP2_Selectable=%s\r\nP3_Selectable=%s\r\nP4_Selectable=%s\r\nP5_Selectable=%s\r\nP6_Selectable=%s\r\nP7_Selectable=%s\r\nP8_Selectable=%s\r\nP9_Selectable=%s\r\nP10_Selectable=%s\r\nP1_Name=%s\r\nP2_Name=%s\r\nP3_Name=%s\r\nP4_Name=%s\r\nP5_Name=%s\r\nP6_Name=%s\r\nP7_Name=%s\r\nP8_Name=%s\r\nP9_Name=%s\r\nP10_Name=%s\r\n", w331, w330, w329, w328, w327, w326, w325, w324, w323, w322, w317, w316, w315, w314, w313, w312, w311, w310, w309, w308) -> (resulting string=w354:string)  [unwired: 2 in, 1 out]
    }
    frame 9 {
      # "SET_PULSE_AMPLITUDE"
      n169 = Array To Cluster(array=w368) -> (cluster=w367:T4)
      n170 = Unbundle By Name(w367) -> ("DATA[0]"=w366:u8)
      n171 = Format Into String(format string="PulseAmplitudeStepIndex=%d\r\n", w366) -> (resulting string=w369:string)  [unwired: 2 in, 1 out]
    }
    frame 10 {
      # "INCREMENT_PULSE_AMPLITUDE"
      n172 = Array To Cluster(array=w374) -> (cluster=w373:T4)
      n173 = Unbundle By Name(w373) -> ("DATA[0]"=w372:u8)
      n174 = Format Into String(format string="PulseVirtualAmplitudeStepIndex=%d\r\n", w372) -> (resulting string=w375:string)  [unwired: 2 in, 1 out]
    }
    frame 11 {
      # "DECREMENT_PULSE_AMPLITUDE"
      n175 = Array To Cluster(array=w380) -> (cluster=w379:T4)
      n176 = Unbundle By Name(w379) -> ("DATA[0]"=w378:u8)
      n177 = Format Into String(format string="PulseVirtualAmplitudeStepIndex=%d\r\n", w378) -> (resulting string=w381:string)  [unwired: 2 in, 1 out]
    }
    frame 12 {
      w399 = "NO"
      w400 = "YES"
      # "GET_PULSE_WIDTHS"
      n178 = Array To Cluster(array=w397) -> (cluster=w398:T6)
      n179 = Unbundle By Name(w398) -> ("DATA[0]"=w396:u8, "DATA[3]"=w385:u8, "DATA[2]"=w384:u8, "DATA[5]"=w387:u8, "DATA[4]"=w386:u8, "DATA[7]"=w389:u8, "DATA[6]"=w388:u8, "DATA[9]"=w391:u8, "DATA[8]"=w390:u8)
      n180 = Join Numbers(hi=w385, lo=w384) -> ((hi.lo)=w395:u16)
      n181 = Join Numbers(hi=w387, lo=w386) -> ((hi.lo)=w394:u16)
      n182 = Join Numbers(hi=w389, lo=w388) -> ((hi.lo)=w393:u16)
      n183 = Join Numbers(hi=w391, lo=w390) -> ((hi.lo)=w392:u16)
      n184 = Number To Boolean Array(number=w396) -> (Boolean array=w410:bool[])
      n185 = Array To Cluster(array=w410) -> (cluster=w409:T2)
      n186 = Unbundle By Name(w409) -> ("Boolean array[0]"=w408:bool, "Boolean array[1]"=w407:bool, "Boolean array[2]"=w406:bool, "Boolean array[3]"=w405:bool)
      n187 = Select(t=w400, s=w408, f=w399) -> (s? t:f=w404:string)
      n188 = Select(t=w400, s=w406, f=w399) -> (s? t:f=w402:string)
      n189 = Select(t=w400, s=w407, f=w399) -> (s? t:f=w403:string)
      n190 = Select(t=w400, s=w405, f=w399) -> (s? t:f=w401:string)
      n191 = Format Into String(format string="PA_Defined=%s\r\nPB_Defined=%s\r\nPC_Defined=%s\r\nPD_Defined=%s\r\nPA_PulseWidth=%d\r\nPB_PulseWidth=%d\r\nPC_PulseWidth=%d\r\nPD_PulseWidth=%d\r\n", w404, w403, w402, w401, w395, w394, w393, w392) -> (resulting string=w411:string)  [unwired: 2 in, 1 out]
    }
    frame 13 {
      # "SET_PULSE_WIDTHS"
    }
    frame 14 {
      # "INCREMENT_PULSE_WIDTH"
      n192 = Array To Cluster(array=w418) -> (cluster=w417:T4)
      n193 = Unbundle By Name(w417) -> ("DATA[0]"=w416:u8)
      n194 = Format Into String(format string="PulseWidth=%d\r\n", w416) -> (resulting string=w419:string)  [unwired: 2 in, 1 out]
    }
    frame 15 {
      # "DECREMENT_PULSE_WIDTH"
      n195 = Array To Cluster(array=w424) -> (cluster=w423:T4)
      n196 = Unbundle By Name(w423) -> ("DATA[0]"=w422:u8)
      n197 = Format Into String(format string="PulseWidth=%d\r\n", w422) -> (resulting string=w425:string)  [unwired: 2 in, 1 out]
    }
    frame 16 {
      # "GET_PROGRAM_FREQUENCY"
      n198 = Array To Cluster(array=w430) -> (cluster=w429:T4)
      n199 = Unbundle By Name(w429) -> ("DATA[0]"=w428:u8)
      n200 = Format Into String(format string="ProgramFrequencyIndex=%d\r\n", w428) -> (resulting string=w431:string)  [unwired: 2 in, 1 out]
    }
    frame 17 {
      # "SET_PROGRAM_FREQUENCY"
    }
    frame 18 {
      # "INCREMENT_PROGRAM_FREQUENCY"
      n201 = Array To Cluster(array=w438) -> (cluster=w437:T4)
      n202 = Unbundle By Name(w437) -> ("DATA[0]"=w436:u8)
      n203 = Format Into String(format string="ProgramFrequencyIndex=%d\r\n", w436) -> (resulting string=w439:string)  [unwired: 2 in, 1 out]
    }
    frame 19 {
      # "DECREMENT_PROGRAM_FREQUENCY"
      n204 = Array To Cluster(array=w444) -> (cluster=w443:T4)
      n205 = Unbundle By Name(w443) -> ("DATA[0]"=w442:u8)
      n206 = Format Into String(format string="ProgramFrequencyIndex=%d\r\n", w442) -> (resulting string=w445:string)  [unwired: 2 in, 1 out]
    }
    frame 20 {
      # "INJECT_EVENT"
    }
    frame 21 {
      # "CHARGING_CONTROL"
      n207 = Array To Cluster(array=w461) -> (cluster=w460:T4)
      n208 = Unbundle By Name(w460) -> ("DATA[0]"=w455:u8, "DATA[1]"=w451:u8)
      n209 = And(x=240, y=w455) -> (x .and. y?=w457:i32)
      n210 = And(x=240, y=w455) -> (x .and. y?=w450:i32)
      n211 = And(x=w455, y=u8 15) -> (x .and. y?=w452:u8)
      n212 = case shown="0, Default" w457 {
        tunnel: ["CHARGE_OFF-0" "CHARGE_PRE_CONDITION-1" "CHARGE_CONSTANT_CURRENT_FAST-2" "CHARGE_CONSTANT_CURRENT_SLOW-3" "CHARGE_COMPLETE-4" "CHARGE_ERROR-5" "CHARGE_CONSTANT_VOLTAGE_FAST-6" "CHARGE_CONSTANT_VOLTAGE_FAST-7"] -> w453
        frame 0, Default {
        }
        frame 16 {
        }
        frame 32 {
        }
        frame 48 {
        }
        frame 64 {
        }
        frame 80 {
        }
        frame 96 {
        }
        frame 112 {
        }
      }
      n213 = case shown="128" w450 {
        tunnel: ["NO" "YES"] -> w454
        frame 0, Default {
        }
        frame 128 {
        }
      }
      n214 = Format Into String(format string="ChargingState=%s\r\nChargeWarning=%s\r\nTemperatureLevel=%d\r\nIPG_ReceivedLevel=%d\r\n", w453, w454, w452, w451) -> (resulting string=w462:string)  [unwired: 2 in, 1 out]
    }
    frame 22 {
      # "GET_XPG_IDENTITY"
      n215 = Array Subset(array=w488, index=0, length=10) -> (w489:u8[])
      n216 = Array Subset(array=w488, index=10 ("length"), length=20) -> (w490:u8[])
      n217 = Array Subset(array=w488, index=30 ("length"), length=10) -> (w491:u8[])
      n218 = Byte Array To String(unsigned byte array=w489) -> (string=w481:string)
      n219 = Byte Array To String(unsigned byte array=w490) -> (string=w480:string)
      n220 = Byte Array To String(unsigned byte array=w491) -> (string=w479:string)
      n221 = Format Into String(format string="ModelNumber=%s\r\nSerialNumber=%s\r\nFirmwareVersion=%s\r\n", w481, w480, w479) -> (resulting string=w476:string)  [unwired: 2 in, 1 out]
      n222 = Search and Replace String(replace all?=TRUE ("replace all? (F)"), input string=w476, search string="\u0000") -> (result string=w475:string)  [unwired: 5 in, 3 out]
    }
    frame 23 {
      # "SET_XPG_IDENTITY"
    }
    frame 24 {
      # "RESTORE_PROGRAM_DEFAULTS"
    }
    frame 25 {
      w513 = "NO"
      w512 = "YES"
      # "GET_PROGRAM_DEFINITION"
      n223 = Index Array(array=w499, index=0) -> (element=w500:u8)
      n224 = Index Array(array=w499, index=2) -> (element=w534:u8)
      n225 = Index Array(array=w499, index=3) -> (element=w532:u8)
      n226 = Index Array(array=w499, index=28) -> (element=w504:u8)
      n227 = Index Array(array=w499, index=29) -> (element=w510:u8)
      n228 = for {
        N: 4 -> [_]
        tunnel: w499 -> [w591]
        shift-right: [w585] -> w503
        shift-left: "" -> [w586]
        i -> [w540]
        w550 = 8 ("index")
        w590 = 54 ("length")
        n229 = Multiply(x=w540, y=w590) -> (x*y=w588:i32)
        n230 = Add(x=30 ("index"), y=w588) -> (x+y=w589:i32)
        n231 = Array Subset(array=w591, index=w589, length=w590) -> (w547:u8[])
        n232 = case shown="3" w540 {
          tunnel: ["\r\n-- PULSE PA --\r\nPulseNamePA=%s\r\nAmplitudeLowLimitPA=%d\r\nAmplitudeStepPA=%d\r\nAmplitudeStepIndexPA=%d\r\nPulseWidthLowLimitPA=%d\r\nPulseWidthHighLimitPA=%d\r\nPulseWidthPA=%d\r\n%s" ("format string") "\r\n-- PULSE PB --\r\nPulseNamePB=%s\r\nAmplitudeLowLimitPB=%d\r\nAmplitudeStepPB=%d\r\nAmplitudeStepIndexPB=%d\r\nPulseWidthLowLimitPB=%d\r\nPulseWidthHighLimitPB=%d\r\nPulseWidthPB=%d\r\n%s" ("format string") "\r\n-- PULSE PC --\r\nPulseNamePC=%s\r\nAmplitudeLowLimitPC=%d\r\nAmplitudeStepPC=%d\r\nAmplitudeStepIndexPC=%d\r\nPulseWidthLowLimitPC=%d\r\nPulseWidthHighLimitPC=%d\r\nPulseWidthPC=%d\r\n%s" ("format string") "\r\n-- PULSE PD --\r\nPulseNamePD=%s\r\nAmplitudeLowLimitPD=%d\r\nAmplitudeStepPD=%d\r\nAmplitudeStepIndexPD=%d\r\nPulseWidthLowLimitPD=%d\r\nPulseWidthHighLimitPD=%d\r\nPulseWidthPD=%d\r\n%s" ("format string")] -> w582
          frame 0, Default {
          }
          frame 1 {
          }
          frame 2 {
          }
          frame 3 {
          }
        }
        n233 = Array Subset(array=w547, index=28, length=26) -> (w544:u8[])
        n234 = Array To Cluster(array=w547) -> (cluster=w579:T7)
        n235 = Unbundle By Name(w579) -> ("[16]"=w576:u8, "[17]"=w575:u8, "[18]"=w571:u8, "[19]"=w572:u8, "[20]"=w566:u8, "[21]"=w565:u8, "[22]"=w560:u8, "[23]"=w559:u8, "[24]"=w551:u8, "[25]"=w552:u8, "[26]"=w554:u8, "[27]"=w553:u8)
        n236 = Array Subset(array=w547, index=0, length=16) -> (w581:u8[])
        n237 = To Unsigned Word Integer(number=w575) -> (unsigned 16bit integer=w578:u16)
        n238 = To Unsigned Word Integer(number=w572) -> (unsigned 16bit integer=w574:u16)
        n239 = To Word Integer(number=w565) -> (16bit integer=w568:i16)
        n240 = To Unsigned Word Integer(number=w559) -> (unsigned 16bit integer=w563:u16)
        n241 = To Unsigned Word Integer(number=w552) -> (unsigned 16bit integer=w558:u16)
        n242 = To Unsigned Word Integer(number=w553) -> (unsigned 16bit integer=w556:u16)
        n243 = Byte Array To String(unsigned byte array=w581) -> (string=w580:string)
        n244 = Logical Shift(y=w550, x=w578) -> (x << y=w577:u16)
        n245 = Logical Shift(y=w550, x=w574) -> (x << y=w573:u16)
        n246 = Logical Shift(y=w550, x=w568) -> (x << y=w567:i16)
        n247 = Logical Shift(y=w550, x=w563) -> (x << y=w562:u16)
        n248 = Logical Shift(y=w550, x=w558) -> (x << y=w557:u16)
        n249 = Logical Shift(y=w550, x=w556) -> (x << y=w555:u16)
        n250 = Add(x=w576, y=w577) -> (x+y=w570:u16)
        n251 = Add(x=w571, y=w573) -> (x+y=w569:u16)
        n252 = Add(x=w566, y=w567) -> (x+y=w564:i16)
        n253 = Add(x=w560, y=w562) -> (x+y=w561:u16)
        n254 = Add(x=w551, y=w557) -> (x+y=w549:u16)
        n255 = Add(x=w554, y=w555) -> (x+y=w548:u16)
        n256 = for {
          N: 26 -> [_]
          tunnel: w544 -> [w603] mode=indexing
          shift-right: [w601] -> w542
          shift-left: "" -> [w602]
          tunnel: w540 -> [w596]
          i -> [w599]
          n257 = case shown="1" w596 {
            tunnel: ["ElectrodeAmpPercentPA[CH%02d]=%d\\r\\n" ("format string") "ElectrodeAmpPercentPB[CH%02d]=%d\\r\\n" ("format string") "ElectrodeAmpPercentPC[CH%02d]=%d\\r\\n" ("format string") "ElectrodeAmpPercentPD[CH%02d]=%d\\r\\n" ("format string")] -> w600
            frame 0, Default {
            }
            frame 1 {
            }
            frame 2 {
            }
            frame 3 {
            }
          }
          n258 = To Byte Integer(number=w603) -> (8bit integer=w597:i8)
          n259 = Increment(x=w599) -> (x+1=w598:i32)
          n260 = Format Into String(format string=w600, initial string=w602, w598, w597) -> (resulting string=w601:string)  [unwired: 1 in, 1 out]
        }
        n261 = Format Into String(format string=w582, initial string=w586, w580, w570, w569, w564, w561, w549, w548, w542) -> (resulting string=w585:string)  [unwired: 1 in, 1 out]
      }
      n262 = Array Subset(array=w499, index=4, length=16) -> (w531:u8[])
      n263 = Array Subset(array=w499, index=20, length=8) -> (w526:u8[])
      n264 = Number To Boolean Array(number=w510) -> (Boolean array=w519:bool[])
      n265 = Greater Than 0?(x=w534) -> (x > 0?=w522:bool)
      n266 = Greater Than 0?(x=w532) -> (x > 0?=w524:bool)
      n267 = Byte Array To String(unsigned byte array=w531) -> (string=w530:string)
      n268 = Array To Cluster(array=w519) -> (cluster=w518:T2)
      n269 = case shown="True" w522 {
        tunnel: ["NO" "YES"] -> w521
        frame False {
        }
        frame True {
        }
      }
      n270 = call <vilib>:"Trim Whitespace.vi"("string"=w530) -> ("trimmed string"=w498:string)  [unwired: 1 in]
      n271 = Unbundle By Name(w518) -> ("Boolean array[0]"=w517:bool, "Boolean array[1]"=w516:bool, "Boolean array[2]"=w515:bool, "Boolean array[3]"=w514:bool)
      n272 = case shown="False" w524 {
        tunnel: ["NO" "YES"] -> w523
        frame False {
        }
        frame True {
        }
      }
      n273 = for {
        shift-right: [w616] -> w525
        shift-left: "" -> [w617]
        tunnel: w526 -> [w618] mode=indexing
        i -> [w613]
        w614 = 8
        n274 = Multiply(x=w614, y=w613) -> (x*y=w612:i32)
        n275 = for {
          N: w614 -> [_]
          shift-right: [w625] -> w615
          shift-left: "" -> [w627]
          tunnel: w618 -> [w628]
          tunnel: w612 -> [w622]
          i -> [w623]
          n276 = Negate(x=w623) -> (-x=w629:i32)
          n277 = Add(x=w622, y=w623) -> (x+y=w621:i32)
          n278 = Logical Shift(y=w629, x=w628) -> (x << y=w630:u8)
          n279 = And(x=u8 1 ("width (-)"), y=w630) -> (x .and. y?=w620:u8)
          n280 = case shown="0, Default" w620 {
            tunnel: ["NO" "YES"] -> w624
            frame 0, Default {
            }
            frame 1 {
            }
          }
          n281 = Format Into String(format string="ProgramFreqTable[%02d]Allowed=%s\\r\\n", initial string=w627, w621, w624) -> (resulting string=w625:string)  [unwired: 1 in, 1 out]
        }
        n282 = Concatenate Strings(w617, w615) -> (w616:string)
      }
      n283 = Select(t=w512, s=w517, f=w513) -> (s? t:f=w509:string)
      n284 = Select(t=w512, s=w515, f=w513) -> (s? t:f=w507:string)
      n285 = Select(t=w512, s=w516, f=w513) -> (s? t:f=w508:string)
      n286 = Select(t=w512, s=w514, f=w513) -> (s? t:f=w506:string)
      n287 = Format Into String(format string="ProgramNumber=%d\r\nProgramDefined=%s\r\nProgramDisabled=%s\r\nProgramName=%s\r\n%sProgramFrequencyIndex=%d\r\nPA_Defined=%s\r\nPB_Defined=%s\r\nPC_Defined=%s\r\nPD_Defined=%s\r\n%s", w500, w521, w523, w498, w525, w504, w509, w508, w507, w506, w503) -> (resulting string=w538:string)  [unwired: 2 in, 1 out]
    }
    frame 26 {
      # "SET_PROGRAM_DEFINITION"
    }
    frame 27 {
      # "GET_PROGRAM_CONSTANTS"
      n288 = for {
        N: 64 -> [_]
        shift-right: [w658] -> w637
        shift-left: "" -> [w659]
        tunnel: w638 -> [w655]
        i -> [w653]
        w652 = 2 ("index")
        n289 = Multiply(x=w653, y=w652) -> (x*y=w654:i32)
        n290 = Add(x=w654, y=w652) -> (x+y=w651:i32)
        n291 = Array Subset(array=w655, index=w651, length=2) -> (w650:u8[])
        n292 = Array To Cluster(array=w650) -> (cluster=w649:cluster{"[0]":u8, "[1]":u8})
        n293 = Unbundle(w649) -> ("[0]"=w645:u8, "[1]"=w644:u8)
        n294 = To Unsigned Word Integer(number=w644) -> (unsigned 16bit integer=w648:u16)
        n295 = Logical Shift(y=i8 8, x=w648) -> (x << y=w646:u16)
        n296 = Add(x=w645, y=w646) -> (x+y=w643:u16)
        n297 = Format Into String(format string="ProgramFrequencies[%02d]=%d\r\n", initial string=w659, w653, w643) -> (resulting string=w658:string)  [unwired: 1 in, 1 out]
      }
      n298 = Format Into String(format string="%s", w637) -> (resulting string=w641:string)  [unwired: 2 in, 1 out]
    }
    frame 28 {
      # "SET_PROGRAM_CONSTANTS"
    }
    frame 29 {
      w671 = "NO"
      w672 = "YES"
      # "Convert MS DateTime\nto LV DateTime"
      # "GET_CONFIGURABLE_DEVICE_PARAMETERS"
      n299 = Array To Cluster(array=w665) -> (cluster=w695:T8)
      n300 = Unbundle By Name(w695) -> ("DATA[0]"=w729:u8, "DATA[1]"=w727:u8, "DATA[2]"=w725:u8, "DATA[3]"=w724:u8, "DATA[4]"=w723:u8, "DATA[5]"=w720:u8, "DATA[6]"=w719:u8, "DATA[7]"=w718:u8, "DATA[8]"=w717:u8, "DATA[9]"=w714:u8, "DATA[10]"=w713:u8, "DATA[11]"=w712:u8)
      n301 = Unbundle By Name(w695) -> ("DATA[42]"=w692:u8, "DATA[43]"=w691:u8, "DATA[44]"=w688:u8, "DATA[45]"=w687:u8, "DATA[46]"=w676:u8)
      n302 = Index Array(array=w665, index=56) -> (element=w664:u8)
      n303 = Array Subset(array=w665, index=48, length=8) -> (w702:u8[])
      n304 = Array Subset(array=w665, index=12, length=30) -> (w697:u8[])
      n305 = for {
        tunnel: w702 -> [w739] mode=indexing
        shift-right: [w733] -> w707
        shift-left: u64 0 ("y") -> [w734]
        tunnel: i8 8 ("y") -> [w737]
        i -> [w738]
        n306 = To Unsigned Quad Integer(1:w739) -> (0:w732:u64)
        n307 = Multiply(x=w737, y=w738) -> (x*y=w736:i32)
        n308 = Logical Shift(y=w736, x=w732) -> (x << y=w735:u64)
        n309 = Add(x=w734, y=w735) -> (x+y=w733:u64)
      }
      n310 = Greater Than 0?(x=w729) -> (x > 0?=w728:bool)
      n311 = Greater Than 0?(x=w723) -> (x > 0?=w722:bool)
      n312 = Greater Than 0?(x=w717) -> (x > 0?=w716:bool)
      n313 = Byte Array To String(unsigned byte array=w697) -> (string=w696:string)
      n314 = To Unsigned Word Integer(number=w691) -> (unsigned 16bit integer=w694:u16)
      n315 = Number To Boolean Array(number=w687) -> (Boolean array=w685:bool[])
      n316 = Number To Boolean Array(number=w676) -> (Boolean array=w677:bool[])
      n317 = Logical Shift(y=i8 8, x=w694) -> (x << y=w693:u16)
      n318 = Array To Cluster(array=w685) -> (cluster=w686:T2)
      n319 = Array To Cluster(array=w677) -> (cluster=w678:T2)
      n320 = Add(x=w692, y=w693) -> (x+y=w689:u16)
      n321 = Unbundle By Name(w686) -> ("Boolean array[0]"=w683:bool, "Boolean array[1]"=w684:bool, "Boolean array[2]"=w681:bool)
      n322 = Unbundle By Name(w678) -> ("Boolean array[0]"=w673:bool, "Boolean array[1]"=w675:bool, "Boolean array[2]"=w674:bool)
      n323 = Multiply(x=u64 1904 ("y"), y=u64 31556926) -> (x*y=w705:u64)
      n324 = Quotient & Remainder(x=w707, y=u64 10000000) -> (floor(x/y)=w663:u64)  [unwired: 1 out]
      n325 = Subtract(x=w663, y=w705) -> (x-y=w703:u64)
      n326 = Format Date/Time String(seconds (now)=w703, UTC format=FALSE) -> (date/time string=w667:string)  [unwired: 1 in]
      n327 = Select(t=w672, s=w722, f=w671) -> (s? t:f=w721:string)
      n328 = Select(t=w672, s=w683, f=w671) -> (s? t:f=w682:string)
      n329 = Select(t=w672, s=w681, f=w671) -> (s? t:f=w679:string)
      n330 = Select(t=w672, s=w675, f=w671) -> (s? t:f=w669:string)
      n331 = Select(t=w672, s=w728, f=w671) -> (s? t:f=w726:string)
      n332 = Select(t=w672, s=w716, f=w671) -> (s? t:f=w715:string)
      n333 = Select(t=w672, s=w684, f=w671) -> (s? t:f=w680:string)
      n334 = Select(t=w672, s=w673, f=w671) -> (s? t:f=w670:string)
      n335 = Select(t=w672, s=w674, f=w671) -> (s? t:f=w668:string)
      n336 = Format Into String(format string="PPC_Enabled=%s\r\nPPC_EXID[0]=0x%02x\r\nPPC_EXID[1]=0x%02x\r\nPPC_EXID[2]=0x%02x\r\nPOP1_Enabled=%s\r\nPOP1_EXID[0]=0x%02x\r\nPOP1_EXID[1]=0x%02x\r\nPOP1_EXID[2]=0x%02x\r\nPOP2_Enabled=%s\r\nPOP2_EXID[0]=0x%02x\r\nPOP2_EXID[1]=0x%02x\r\nPOP2_EXID[2]=0x%02x\r\nPPC_Text=%s\r\nPulseWidthStep=%d\r\nAmplitudeSteps=%d\r\nPPC_AllowIndividualPulseAmplMod=%s\r\nPPC_AllowIndividualPulseWidthMod=%s\r\nPPC_AllowProgramFreqMod=%s\r\nIPG_MagnetOptions_Behavior_A_Enabled=%s\r\nIPG_MagnetOptions_Behavior_B_Enabled=%s\r\nIPG_MagnetOptions_Behavior_C_Enabled=%s\r\nImplantDateTime=%s\r\nReplacementIntervalMonths=%d\r\n", w726, w727, w725, w724, w721, w720, w719, w718, w715, w714, w713, w712, w696, w689, w688, w682, w680, w679, w670, w669, w668, w667, w664) -> (resulting string=w730:string)  [unwired: 2 in, 1 out]
    }
    frame 30 {
      # "SET_CONFIGURABLE_DEVICE_PARAMETERS"
    }
    frame 31 {
      w751 = "NO"
      w750 = "YES"
      w796 = i8 8 ("y")
      # "GET_PULSE_CONSTANTS"
      n337 = Array To Cluster(array=w817) -> (cluster=w818:T9)
      n338 = Unbundle By Name(w818) -> ("DATA[0]"=w795:u8, "DATA[1]"=w775:u8, "DATA[2]"=w794:u8, "DATA[3]"=w743:u8, "DATA[4]"=w793:u8, "DATA[5]"=w776:u8, "DATA[6]"=w792:u8, "DATA[7]"=w777:u8, "DATA[8]"=w791:u8, "DATA[9]"=w778:u8, "DATA[10]"=w790:u8, "DATA[11]"=w779:u8, "DATA[12]"=w789:u8, "DATA[13]"=w780:u8, "DATA[14]"=w788:u8, "DATA[15]"=w781:u8, "DATA[16]"=w787:u8, "DATA[17]"=w782:u8, "DATA[18]"=w786:u8, "DATA[19]"=w783:u8, "DATA[20]"=w785:u8, "DATA[21]"=w784:u8, "DATA[22]"=w749:u8, "DATA[23]"=w748:u8)
      n339 = To Unsigned Word Integer(number=w775) -> (unsigned 16bit integer=w820:u16)
      n340 = To Unsigned Word Integer(number=w743) -> (unsigned 16bit integer=w816:u16)
      n341 = To Unsigned Word Integer(number=w776) -> (unsigned 16bit integer=w814:u16)
      n342 = To Unsigned Word Integer(number=w777) -> (unsigned 16bit integer=w812:u16)
      n343 = To Unsigned Word Integer(number=w778) -> (unsigned 16bit integer=w810:u16)
      n344 = To Unsigned Word Integer(number=w779) -> (unsigned 16bit integer=w808:u16)
      n345 = To Unsigned Word Integer(number=w780) -> (unsigned 16bit integer=w806:u16)
      n346 = To Unsigned Word Integer(number=w781) -> (unsigned 16bit integer=w804:u16)
      n347 = To Unsigned Word Integer(number=w782) -> (unsigned 16bit integer=w802:u16)
      n348 = To Unsigned Word Integer(number=w783) -> (unsigned 16bit integer=w800:u16)
      n349 = To Unsigned Word Integer(number=w784) -> (unsigned 16bit integer=w798:u16)
      n350 = Logical Shift(y=w796, x=w820) -> (x << y=w819:u16)
      n351 = Logical Shift(y=w796, x=w816) -> (x << y=w815:u16)
      n352 = Logical Shift(y=w796, x=w814) -> (x << y=w813:u16)
      n353 = Logical Shift(y=w796, x=w812) -> (x << y=w811:u16)
      n354 = Logical Shift(y=w796, x=w810) -> (x << y=w809:u16)
      n355 = Logical Shift(y=w796, x=w808) -> (x << y=w807:u16)
      n356 = Logical Shift(y=w796, x=w806) -> (x << y=w805:u16)
      n357 = Logical Shift(y=w796, x=w804) -> (x << y=w803:u16)
      n358 = Logical Shift(y=w796, x=w802) -> (x << y=w801:u16)
      n359 = Logical Shift(y=w796, x=w800) -> (x << y=w799:u16)
      n360 = Logical Shift(y=w796, x=w798) -> (x << y=w797:u16)
      n361 = Add(x=w795, y=w819) -> (x+y=w774:u16)
      n362 = Add(x=w794, y=w815) -> (x+y=w773:u16)
      n363 = Add(x=w793, y=w813) -> (x+y=w772:u16)
      n364 = Add(x=w792, y=w811) -> (x+y=w771:u16)
      n365 = Add(x=w791, y=w809) -> (x+y=w770:u16)
      n366 = Add(x=w790, y=w807) -> (x+y=w769:u16)
      n367 = Add(x=w789, y=w805) -> (x+y=w768:u16)
      n368 = Add(x=w788, y=w803) -> (x+y=w767:u16)
      n369 = Add(x=w787, y=w801) -> (x+y=w766:u16)
      n370 = Add(x=w786, y=w799) -> (x+y=w765:u16)
      n371 = Add(x=w785, y=w797) -> (x+y=w752:u16)
      n372 = Number To Boolean Array(number=w765) -> (Boolean array=w764:bool[])
      n373 = Array To Cluster(array=w764) -> (cluster=w763:T10)
      n374 = Unbundle By Name(w763) -> ("Boolean array[0]"=w762:bool, "Boolean array[1]"=w761:bool, "Boolean array[2]"=w760:bool, "Boolean array[3]"=w755:bool, "Boolean array[4]"=w754:bool)
      n375 = Greater Than 0?(x=w749) -> (x > 0?=w747:bool)
      n376 = Greater Than 0?(x=w748) -> (x > 0?=w746:bool)
      n377 = Select(t=w750, s=w762, f=w751) -> (s? t:f=w759:string)
      n378 = Select(t=w750, s=w760, f=w751) -> (s? t:f=w757:string)
      n379 = Select(t=w750, s=w754, f=w751) -> (s? t:f=w753:string)
      n380 = Select(t=w750, s=w746, f=w751) -> (s? t:f=w744:string)
      n381 = Select(t=w750, s=w761, f=w751) -> (s? t:f=w758:string)
      n382 = Select(t=w750, s=w755, f=w751) -> (s? t:f=w756:string)
      n383 = Select(t=w750, s=w747, f=w751) -> (s? t:f=w745:string)
      n384 = Format Into String(format string="PassiveInterphaseDelay=%d\r\nPassiveRecoveryWidth=%d\r\nPassiveRecoveryHoldoff=%d\r\nPassiveCBCWidth=%d\r\nPassiveCBCHoldoff=%d\r\nActiveInterphaseDelay=%d\r\nActiveRecoveryHoldoff=%d\r\nActiveCBCWidth=%d\r\nActiveCBCHoldoff=%d\r\nKrec[1]Enabled=%s\r\nKrec[2]Enabled=%s\r\nKrec[3]Enabled=%s\r\nKrec[4]Enabled=%s\r\nKrec[5]Enabled=%s\r\nIncrementLockoutMsecs=%d\r\nStimPhasePSDisableActive=%s\r\nUncontrolledSourceSinkEnabled=%s\r\n", w774, w773, w772, w771, w770, w769, w768, w767, w766, w759, w758, w757, w756, w753, w752, w745, w744) -> (resulting string=w821:string)  [unwired: 2 in, 1 out]
    }
    frame 32 {
      # "SET_PULSE_CONSTANTS"
    }
    frame 33 {
      # "GET_LEAD_LIMITS"
      n385 = for {
        N: 26 -> [_]
        shift-right: [w871] -> w826
        shift-left: "" -> [w872]
        tunnel: w828 -> [w868]
        i -> [w866]
        n386 = Multiply(x=w866, y=2 ("index")) -> (x*y=w867:i32)
        n387 = Add(x=w867, y=52) -> (x+y=w864:i32)
        n388 = Array Subset(array=w868, index=w864, length=2) -> (w863:u8[])
        n389 = Increment(x=w866) -> (x+1=w854:i32)
        n390 = Array To Cluster(array=w863) -> (cluster=w862:cluster{"[0]":u8, "[1]":u8})
        n391 = Unbundle(w862) -> ("[0]"=w858:u8, "[1]"=w857:u8)
        n392 = To Unsigned Word Integer(number=w857) -> (unsigned 16bit integer=w861:u16)
        n393 = Logical Shift(y=i8 8, x=w861) -> (x << y=w859:u16)
        n394 = Add(x=w858, y=w859) -> (x+y=w856:u16)
        n395 = Format Into String(format string="chargeLimit[%02d]=%d\r\n", initial string=w872, w854, w856) -> (resulting string=w871:string)  [unwired: 1 in, 1 out]
      }
      n396 = for {
        N: 26 -> [_]
        shift-right: [w852] -> w827
        shift-left: "" -> [w853]
        tunnel: w828 -> [w849]
        i -> [w847]
        n397 = Multiply(x=w847, y=2 ("index")) -> (x*y=w848:i32)
        n398 = Add(x=w848, y=0) -> (x+y=w845:i32)
        n399 = Array Subset(array=w849, index=w845, length=2) -> (w844:u8[])
        n400 = Increment(x=w847) -> (x+1=w835:i32)
        n401 = Array To Cluster(array=w844) -> (cluster=w843:cluster{"[0]":u8, "[1]":u8})
        n402 = Unbundle(w843) -> ("[0]"=w839:u8, "[1]"=w838:u8)
        n403 = To Unsigned Word Integer(number=w838) -> (unsigned 16bit integer=w842:u16)
        n404 = Logical Shift(y=i8 8, x=w842) -> (x << y=w840:u16)
        n405 = Add(x=w839, y=w840) -> (x+y=w837:u16)
        n406 = Format Into String(format string="currentLimit[%02d]=%d\r\n", initial string=w853, w835, w837) -> (resulting string=w852:string)  [unwired: 1 in, 1 out]
      }
      n407 = Format Into String(format string="%s%s", w827, w826) -> (resulting string=w833:string)  [unwired: 2 in, 1 out]
    }
    frame 34 {
      # "SET_LEAD_LIMITS"
    }
    frame 35 {
      # "GET_CHANNEL_CALIBRATIONS"
      n408 = Split 1D Array(array=w888, index=2) -> (first subarray=w877:u8[], second subarray=w886:u8[])
      n409 = for {
        N: 26 -> [_]
        shift-right: [w931] -> w885
        shift-left: "" -> [w932]
        tunnel: w886 -> [w928]
        i -> [w926]
        n410 = Multiply(x=w926, y=2 ("index")) -> (x*y=w927:i32)
        n411 = Add(x=w927, y=52) -> (x+y=w924:i32)
        n412 = Array Subset(array=w928, index=w924, length=2) -> (w923:u8[])
        n413 = Increment(x=w926) -> (x+1=w914:i32)
        n414 = Array To Cluster(array=w923) -> (cluster=w922:cluster{"[0]":u8, "[1]":u8})
        n415 = Unbundle(w922) -> ("[0]"=w918:u8, "[1]"=w917:u8)
        n416 = To Unsigned Word Integer(number=w917) -> (unsigned 16bit integer=w921:u16)
        n417 = Logical Shift(y=i8 8, x=w921) -> (x << y=w919:u16)
        n418 = Add(x=w918, y=w919) -> (x+y=w916:u16)
        n419 = Format Into String(format string="channelCalSinking[%02d]=%d\r\n", initial string=w932, w914, w916) -> (resulting string=w931:string)  [unwired: 1 in, 1 out]
      }
      n420 = for {
        N: 26 -> [_]
        shift-right: [w912] -> w884
        shift-left: "" -> [w913]
        tunnel: w886 -> [w909]
        i -> [w907]
        n421 = Multiply(x=w907, y=2 ("index")) -> (x*y=w908:i32)
        n422 = Add(x=w908, y=0) -> (x+y=w905:i32)
        n423 = Array Subset(array=w909, index=w905, length=2) -> (w904:u8[])
        n424 = Increment(x=w907) -> (x+1=w895:i32)
        n425 = Array To Cluster(array=w904) -> (cluster=w903:cluster{"[0]":u8, "[1]":u8})
        n426 = Unbundle(w903) -> ("[0]"=w899:u8, "[1]"=w898:u8)
        n427 = To Unsigned Word Integer(number=w898) -> (unsigned 16bit integer=w902:u16)
        n428 = Logical Shift(y=i8 8, x=w902) -> (x << y=w900:u16)
        n429 = Add(x=w899, y=w900) -> (x+y=w897:u16)
        n430 = Format Into String(format string="channelCalSourcing[%02d]=%d\r\n", initial string=w913, w895, w897) -> (resulting string=w912:string)  [unwired: 1 in, 1 out]
      }
      n431 = Array To Cluster(array=w877) -> (cluster=w883:cluster{"[0]":u8, "[1]":u8})
      n432 = Unbundle(w883) -> ("[0]"=w879:u8, "[1]"=w878:u8)
      n433 = To Unsigned Word Integer(number=w878) -> (unsigned 16bit integer=w882:u16)
      n434 = Logical Shift(y=i8 8, x=w882) -> (x << y=w880:u16)
      n435 = Add(x=w879, y=w880) -> (x+y=w876:u16)
      n436 = Format Into String(format string="Index=%d\r\n%s%s", w876, w884, w885) -> (resulting string=w893:string)  [unwired: 2 in, 1 out]
    }
    frame 36 {
      # "SET_CHANNEL_CALIBRATIONS"
    }
    frame 43 {
      # "GET_STIM_ASIC_HV_CALIBRATIONS"
      n437 = for {
        N: 64 -> [_]
        shift-right: [w958] -> w936
        shift-left: "" -> [w959]
        tunnel: w937 -> [w955]
        i -> [w953]
        n438 = Multiply(x=w953, y=2 ("index")) -> (x*y=w954:i32)
        n439 = Add(x=w954, y=0) -> (x+y=w951:i32)
        n440 = Array Subset(array=w955, index=w951, length=2) -> (w950:u8[])
        n441 = Array To Cluster(array=w950) -> (cluster=w949:cluster{"[0]":u8, "[1]":u8})
        n442 = Unbundle(w949) -> ("[0]"=w945:u8, "[1]"=w944:u8)
        n443 = To Unsigned Word Integer(number=w944) -> (unsigned 16bit integer=w948:u16)
        n444 = Logical Shift(y=i8 8, x=w948) -> (x << y=w946:u16)
        n445 = Add(x=w945, y=w946) -> (x+y=w943:u16)
        n446 = Format Into String(format string="Stim_ASIC_HV_mV_Output[%02d]=%d\r\n", initial string=w959, w953, w943) -> (resulting string=w958:string)  [unwired: 1 in, 1 out]
      }
      n447 = Format Into String(format string="%s", w936) -> (resulting string=w940:string)  [unwired: 2 in, 1 out]
    }
    frame 44 {
      # "SET_STIM_ASIC_HV_CALIBRATIONS"
    }
    frame 47 {
      w962 = 0 ("index")
      # "GET_CP_DATA"
      n448 = Delete From Array(array=w971, length=2, index=w962) -> (deleted portion=w963:u8[], array with subset deleted=w967:u8[])
      n449 = Index Array(array=w963, index=w962) -> (element=w964:u8)
      n450 = Format Into String(format string="CP_Data_Block=%d\r\n", w964) -> (resulting string=w965:string)  [unwired: 2 in, 1 out]
      n451 = for {
        N: 256 -> [_]
        shift-right: [w978] -> w970
        shift-left: w965 -> [w979]
        tunnel: w967 -> [w975] mode=indexing
        tunnel: [w975] -> w969 mode=indexing
        i -> [w976]
        n452 = Format Into String(format string="CP_Data[%03d]=0x%02x\r\n", initial string=w979, w976, w975) -> (resulting string=w978:string)  [unwired: 1 in, 1 out]
      }
      n453 = Format Into String(format string="%s", w970) -> (resulting string=w973:string)  [unwired: 2 in, 1 out]
    }
    frame 48 {
      # "SET_CP_DATA"
    }
    frame 49 {
      # "CLEAR_LOG"
    }
    frame 50 {
      w999 = string[][] [["0", " The null event."], ["1001", " An unintended reset occurred."], ["1002", " A watchdog reset occurred."], ["1003", " An error was detected during a voltage check."], ["1004", " An error was detected during a temperature check."], ["1005", " A timing error was detected during clock verification."], ["1006", " A timing error was detected during pulse cycle verification"], ["1010", " A Stimulation Data Read-back error was detected."], ["1011", " The diagnostic memory check detected corruption of the Stimulation Program Definition."], ["1012", " The diagnostic memory check detected corruption of the Active Stimulation Settings."], ["1013", " The diagnostic memory check detected corruption of the MICS identity information."], ["1014", " The diagnostic memory check detected corruption of the Program Constants."], ["1015", " The diagnostic memory check detected corruption of the Pulse Constants."], ["1016", " The diagnostic memory check detected corruption of the Channel Calibration."], ["1017", " The diagnostic memory check detected corruption of the Lead Information."], ["1018", " The diagnostic memory check detected corruption of the Configurable Device Parameters."], ["1019", " The diagnostic memory check detected corruption of the General Calibration Data."], ["1020", " The Stimulation System trim list is corrupted."], ["1021", " The Power System trim list is corrupted."], ["1022", " The Radio trim list is corrupted."], ["1023", " The Program Data Integrity check failed"], ["1024", " The diagnostic memory check detected corruption of the High Voltage Calibration"], ["1025", " The diagnostic memory check detected corruption of the Background Impedance Parameters"], ["1026", " The diagnostic memory check detected corruption of the Ramp Time"], ["1030", " A Brownout was detected during Stimulation."], ["1040", " The pulse guard tripped."], ["1041", " A stimulation system parity error was detected."], ["1042", " A stimulation system sequencing error"], ["1043", " A stimulation system address error"], ["1044", " A stimulation system register valid error"], ["1045", " A stimulation system write protect error"], ["1050", " The Impedance Measurement diagnostics detected an Open Circuit Condition."], ["1051", " The Background Stimulation Output check detected a Faulty Channel."], ["1052", " The Output Capacitor check detected a Faulty Capacitor."], ["1053", " Background Impedance Measurement failed"], ["1054", " The Check Densities routine failed"], ["1055", " The Stimulation hardware didn't power up or initialize correctly"], ["1056", " Basic Output Check failed"], ["1057", " Diagnostic Output Check failed"], ["1060", " The Thermistor Diagnostic detects a fault in the temperature measurement circuit"], ["1070", " The Log Module detected a corrupt Event Log data structure in this Log"], ["1071", " The software has exceeded its stack limitations"], ["1072", " The software has detected a queue overflow"], ["1080", " Unknown error has been published"], ["1081", " System restarted after coming out of reset"], ["1082", " System restarted after receiving unknown interrupt"], ["1083", " System restarted for unknown reasons"], ["1090", " Test stim range check failed"], ["1091", " Retrieving a program failed"], ["1092", " Stim auto-waveform failed"], ["1093", " Compliance voltage calculation indicates voltage higher than is available"], ["1094", " Stim high voltage DAC initialization failed"], ["1095", " Stim period check failed"], ["1096", " Stim calculated a pulse width - frequency conflict"], ["2001", " Embed timestamp low bytes in log"], ["2002", " Mark location in log"], ["2003", " System is powered up or coming out of a reset"], ["2004", " CP has been connected to the system"], ["2005", " Embed timestamp high bytes in log"], ["2006", " MICS Connection established data includes channel number"], ["2007", " MICS has been disconnected by the software"], ["2008", " MICS has been shutdown"], ["2009", " MICS transmit/receive has been aborted"], ["2010", " MICS driver has been initialized"], ["2011", " MICS connection has been lost"], ["2012", " MICS radio failure"], ["2013", " MICS radio is ready"], ["2014", " MICS link is ready"], ["2016", " MICS MAC Command Timeout"], ["2017", " MICS Watchdog Timeout"], ["2018", " MICS Housekeeping Abort Link"], ["2020", " Charging of the battery has been initiated"], ["2021", " Battery has been charged to full capacity"], ["2022", " Battery charging has been interrupted prior to being fully charged"], ["2023", " Charger has been detected"], ["2024", " Charger has been removed"], ["2025", " Charging has been aborted due to high temperature"], ["2026", " Charging has been aborted due to insufficient voltage rise"], ["2027", " Charging has been aborted due to error"], ["2028", " Charging has been disconnected from the system"], ["2029", " Stimulation was stopped due to low battery"], ["2030", " Stimulation was stopped due to power down"], ["2031", " Stimulation was stopped due to an error"], ["2032", " Charging was stopped due to overvoltage error"], ["2033", " Charging was switched to C8 because of critical temperature"], ["2034", " Charging was switched to the mode specified"], ["2040", " Stimulation was stopped to radio session closing"], ["2041", " Pairing information was changed via radio"], ["2042", " Pairing information was changed via charging system"], ["2050", " Calibration data restored from backup"], ["2051", " Program or Pulse constants data has been repaired"], ["2052", " High Voltage Calibration data was restored from backup"], ["2053", " General Calibration data was restored from backup"], ["2054", " System Information Data was restored from backup copy"], ["2055", " Stimulation configuration trim list data was restored from backup"], ["2056", " Radio configuration trim list data was restored from backup"], ["2057", " Default background impedance parameters have been restored"], ["2058", " Power configuration trim list data was restored from backup"], ["2059", " Configurable device parameters was restored from backup"], ["2060", " Ramp time was restored from backup"], ["2070", " The command received was not supported"], ["2071", " Stimulation was stopped"], ["2072", " Patient stimulation was started"], ["2073", " Trial stimulation was started"], ["2074", " Test stimulation was started"], ["2075", " System was commanded into storage mode"], ["2076", " Patient Program was selected"], ["2077", " Program amplitude was incremented"], ["2078", " Pulse amplitude was incremented"], ["2079", " Program frequency was set"], ["2080", " Active Program Settings were restored to default values"], ["2081", " System was commanded to reset"], ["2082", " Impedance measurement was requested"], ["2083", " Log was requested to be cleared"], ["2084", " Trial Stimulation parameters were modified"], ["2089", " Test Stimulation parameters were modified"], ["2090", " Program amplitude was decremented"], ["2100", " Patient stimulation was started via magnet"], ["2101", " Patient stimulation was stopped via magnet"], ["2102", " System is about the powered down via magnet"], ["2110", " Stimulation is stopped via charging system command"], ["2120", " Error log was read"], ["2121", " Event log was read"], ["2122", " PPC Constants were queried"], ["2123", " Program names were queried"], ["2124", " Program constants were queried"], ["2125", " System Identity information was queried"], ["2126", " General calibration parameters were queried"], ["2127", " Charging went from current mode to voltage mode counter was queried"], ["2128", " Charging was done to completion counter was queried"], ["2129", " Storage mode counter was queried"], ["2130", " Channel calibration values were queried"], ["2131", " High Voltage calibration values were queried"], ["2132", " Trim list values were queried"], ["2133", " Battery diagnostic information was queried"], ["2134", " Background impedance diagnostic information was queried"], ["2135", " Output capacitor check diagnostic information was queried"], ["2136", " Thermistor diagnostic information was queried"], ["2137", " Program definition was queried"], ["2138", " Pulse constants were queried"], ["2139", " Configuration device parameters were queried"], ["2140", " Pulse widths were queried"], ["2141", " Program frequency was queried"], ["2142", " POP Constants were queried"], ["2143", " Lead limits were queried"], ["2144", " Clinician Programmer data was queried"], ["2145", " Ramp Time was queried"], ["2146", " Trial Stimulation parameters were queried"], ["2147", " Program run time was queried"], ["2148", " Direct memory read was performed"], ["2149", " Background impedance parameters were queried"], ["2201", " System Identity Information changed"], ["2202", " General calibration data changed"], ["2203", " Charging mode change counter was reset"], ["2204", " Charging completed counter was reset"], ["2205", " Storage mode counter was reset"], ["2206", " Channel calibration was changed"], ["2207", " High Voltage calibration was changed"], ["2208", " Stimulation configuration trim list was changed"], ["2209", " Radio configuration trim list was changed"], ["2210", " Program definition was changed"], ["2211", " Program constants were changed"], ["2212", " Pulse constants were changed"], ["2213", " Config device parameters were changed"], ["2214", " Lead limits were changed"], ["2215", " Clinician Program data was changed"], ["2216", " Ramp Time was changed"], ["2217", " Program Time was reset"], ["2218", " Direct write to memory was requested"], ["2219", " Background Impedance Parameters were changed"], ["2220", " System Error was detected"], ["2221", " Charging Error was detected"], ["2222", " Power configuration trim list was changed"], ["2300", " Diagnostic log of vrect and temperature during charging"], ["2301", " Diagnostic log of temperature data during charging"], ["2302", " Diagnostic log of battery adc counts during charging"], ["2303", " The MICS ISR was unable to clear an interrupt bit. Data contains (lsb) after processing irq stat2 register after processing irq stat 1 register before processing irq stat 2 register before processing irq stat 1 register (msb)"], ["2304", " The MICS driver failed to write to a register via SPI. Data contains (lsb) read register value written register value register address (msb)"], ["2305", " The MSP430 VLO was calibrated and is running at the specified frequency"], ["2400", " A MICS Command was received token is logged"], ["2401", " A MICS Response was sent token is logged"], ["2402", " A MICS Packet was dumped"], ["2403", " A MICS Command was received from an unpaired programmer"], ["2404", " A MICS Command with an invalid token was received"], ["2405", " A MICS Command was received but the checksum failed"], ["2406", " A MICSPAD Timeout occurred waiting for an intermediate block"], ["2407", " A MICS Session was closed by the MICS PAD"], ["2450", " A byte was received over TETS data has byte"], ["2451", " A valid TETS command was received data has command number"], ["2452", " A response is being sent over TETS"], ["2453", " A byte was sent over TETS data has byte"], ["2454", " TETS command was rejected because message not formatted correctly"], ["2455", " A timeout occurred while sending or receving data bytes"], ["2500", "Debug"], ["", "PULSE_GUARD_MEMORY_ERROR"], ["", "PULSE_GUARD_CLOCK_ERROR"], ["", "PULSE_GUARD_UNKNOWN_ERROR"]]  # Event descriptions from .h file
      # "( Mark's updates )"
      # "READ_LOG"
      n454 = Array To Cluster(array=w1002) -> (cluster=w986:T6)
      n455 = Unbundle By Name(w986) -> ("DATA[0]"=w987:u8, "DATA[1]"=w994:u8, "DATA[7]"=w990:u8, "DATA[6]"=w991:u8, "DATA[5]"=w992:u8, "DATA[4]"=w993:u8)
      n456 = Join Numbers(hi=w990, lo=w991) -> ((hi.lo)=w989:u16)
      n457 = Join Numbers(hi=w992, lo=w993) -> ((hi.lo)=w988:u16)
      n458 = Join Numbers(hi=w989, lo=w988) -> ((hi.lo)=w1000:u32)
      n459 = Array Subset(array=w1002, index=8) -> (w995:u8[])  [unwired: 1 in]
      n460 = for {
        N: w994 -> [_]
        tunnel: w995 -> [w1034]
        tunnel: 10 ("index") -> [w1019]
        shift-right: [w1031] -> w1001
        shift-left: "" -> [w1030]
        tunnel: w999 -> [w1009]
        i -> [w1018]
        n461 = Index Array(array=w1009, index (col) #1=0 ("disabled index (col)"), index (col) #2=1 ("disabled index (col)")) -> (element #1=w1012:string[], element #2=w1005:string[])  [unwired: 2 in]
        n462 = Multiply(x=w1018, y=w1019) -> (x*y=w1014:i32)
        n463 = Array Subset(array=w1034, index=w1014, length=w1019) -> (w1033:u8[])
        n464 = Array To Cluster(array=w1033) -> (cluster=w1032:T11)
        n465 = Unbundle By Name(w1032) -> ("[3]"=w1026:u8, "[2]"=w1025:u8, "[1]"=w1024:u8, "[0]"=w1023:u8, "[5]"=w1016:u8, "[4]"=w1017:u8, "[6]"=w1008:u8, "[7]"=w1021:u8, "[8]"=w1020:u8, "[9]"=w1015:u8)
        n466 = Join Numbers(hi=w1026, lo=w1025) -> ((hi.lo)=w1027:u16)
        n467 = Join Numbers(hi=w1024, lo=w1023) -> ((hi.lo)=w1028:u16)
        n468 = Join Numbers(hi=w1016, lo=w1017) -> ((hi.lo)=w1004:u16)
        n469 = Join Numbers(hi=w1027, lo=w1028) -> ((hi.lo)=w1022:u32)
        n470 = Number To Decimal String(number=w1004) -> (decimal integer string=w1011:string)  [unwired: 1 in]
        n471 = Search 1D Array(1D array=w1012, element=w1011) -> (index of element=w1010:i32)  [unwired: 1 in]
        n472 = Index Array(array=w1005, index=w1010) -> (element=w1007:string)
        n473 = Format Into String(format string="\\r\\nTimestamp=%d\\r\\nEvent=%d\\r\\nDescription=%s\\r\\nEventData[0]=%02x\\r\\nEventData[1]=%02x\\r\\nEventData[2]=%02x\\r\\nEventData[3]=%02x\\r\\n", initial string=w1030, w1022, w1004, w1007, w1008, w1021, w1020, w1015) -> (resulting string=w1031:string)  [unwired: 1 in, 1 out]
      }
      n474 = Format Into String(format string="LogNum=%d\r\nCount=%d\r\nSerial=%d\r\n%s", w987, w994, w1000, w1001) -> (resulting string=w1003:string)  [unwired: 2 in, 1 out]
    }
    frame 51 {
      # "APPEND_LOG"
      n475 = Array To Cluster(array=w1037) -> (cluster=w1038:T6)
      n476 = disable-structure shown="Enabled" {
        disable-tunnel: w1038 -> [w1048 w1050]
        disable-tunnel: [w1041 w1049] -> w1036
        frame Enabled {
          n477 = Unbundle By Name(w1048) -> ("DATA[3]"=w1047:u8, "DATA[2]"=w1046:u8, "DATA[1]"=w1045:u8, "DATA[0]"=w1044:u8)
          n478 = Join Numbers(hi=w1047, lo=w1046) -> ((hi.lo)=w1043:u16)
          n479 = Join Numbers(hi=w1045, lo=w1044) -> ((hi.lo)=w1042:u16)
          n480 = Join Numbers(hi=w1043, lo=w1042) -> ((hi.lo)=w1041:u32)
        }
        frame Disabled {
          n481 = Unbundle By Name(w1050) -> ("DATA[0]"=w1049:u8)
        }
      }
      n482 = Format Into String(format string="Serial=%d\r\n", w1036) -> (resulting string=w1039:string)  [unwired: 2 in, 1 out]
    }
    frame 52 {
      # "GET_PATIENT_PROGRAM_RUN-TIME"
      n483 = Array To Cluster(array=w1060) -> (cluster=w1061:T6)
      n484 = Unbundle By Name(w1061) -> ("DATA[0]"=w1059:u8, "DATA[5]"=w1056:u8, "DATA[4]"=w1055:u8, "DATA[3]"=w1054:u8, "DATA[2]"=w1053:u8)
      n485 = Join Numbers(hi=w1056, lo=w1055) -> ((hi.lo)=w1058:u16)
      n486 = Join Numbers(hi=w1054, lo=w1053) -> ((hi.lo)=w1057:u16)
      n487 = Join Numbers(hi=w1058, lo=w1057) -> ((hi.lo)=w1052:u32)
      n488 = Format Into String(format string="patientProgramNumber=%d\r\npatientProgramRunTime=%d\r\n", w1059, w1052) -> (resulting string=w1062:string)  [unwired: 2 in, 1 out]
    }
    frame 84 {
      # "GET_LOG_RANGE"
      n489 = Array To Cluster(array=w1081) -> (cluster=w1082:T6)
      n490 = Unbundle By Name(w1082) -> ("DATA[0]"=w1072:u8, "DATA[7]"=w1068:u8, "DATA[6]"=w1069:u8, "DATA[5]"=w1070:u8, "DATA[4]"=w1071:u8, "DATA[11]"=w1064:u8, "DATA[10]"=w1065:u8, "DATA[9]"=w1066:u8, "DATA[8]"=w1067:u8)  [unwired: 3 out]
      n491 = Join Numbers(hi=w1068, lo=w1069) -> ((hi.lo)=w1078:u16)
      n492 = Join Numbers(hi=w1070, lo=w1071) -> ((hi.lo)=w1079:u16)
      n493 = Join Numbers(hi=w1064, lo=w1065) -> ((hi.lo)=w1077:u16)
      n494 = Join Numbers(hi=w1066, lo=w1067) -> ((hi.lo)=w1076:u16)
      n495 = Join Numbers(hi=w1078, lo=w1079) -> ((hi.lo)=w1075:u32)
      n496 = Join Numbers(hi=w1077, lo=w1076) -> ((hi.lo)=w1074:u32)
      n497 = Subtract(x=w1074, y=w1075) -> (x-y=w1073:u32)
      n498 = Format Into String(format string="LogNum=%d\r\nminSerialNum=%d\r\nmaxSerialNum=%d\r\nnumEntries=%d\r\n", w1072, w1075, w1074, w1073) -> (resulting string=w1083:string)  [unwired: 2 in, 1 out]
    }
    frame 53 {
      # "SET_PATIENT_PROGRAM_RUN-TIME"
    }
    frame 54 {
      # "IMPEDANCE_MEASUREMENT"
      n499 = Array To Cluster(array=w1091) -> (cluster=w1094:T6)
      n500 = Unbundle By Name(w1094) -> ("DATA[0]"=w1093:u8, "DATA[1]"=w1092:u8, "DATA[3]"=w1090:u8, "DATA[2]"=w1089:u8)
      n501 = Join Numbers(hi=w1090, lo=w1089) -> ((hi.lo)=w1088:u16)
      n502 = Format Into String(format string="channel_A=%d\r\nchannel_B=%d\r\nimpedanceReading=%d\r\n", w1093, w1092, w1088) -> (resulting string=w1095:string)  [unwired: 2 in, 1 out]
    }
    frame 55 {
      # "ENTER_STORAGE_MODE"
    }
    frame 56 {
      # "Echo Short"
      n503 = Array Subset(array=w1103, index=0, length=8) -> (w1101:u8[])
      n504 = Byte Array To String(unsigned byte array=w1101) -> (string=w1100:string)
      n505 = Format Into String(format string="%s", w1100) -> (resulting string=w1105:string)  [unwired: 2 in, 1 out]
    }
    frame 57 {
      # "Echo Long"
      n506 = Array Subset(array=w1109, index=0, length=256) -> (w1110:u8[])
      n507 = Byte Array To String(unsigned byte array=w1110) -> (string=w1108:string)
      n508 = Format Into String(format string="%s", w1108) -> (resulting string=w1113:string)  [unwired: 2 in, 1 out]
    }
    frame 58 {
      # "GET_GENERAL_CALIBRATION"
      n509 = Array Subset(array=w1131, index=0, length=30) -> (w1160:u8[])
      n510 = Array Subset(array=w1131, index=30, length=24) -> (w1130:u8[])
      n511 = Array Subset(array=w1131, index=54, length=30) -> (w1155:u8[])
      n512 = Array Subset(array=w1131, index=84, length=18) -> (w1152:u8[])
      n513 = Array Subset(array=w1131, index=92, length=18) -> (w1150:u8[])
      n514 = Index Array(array=w1131, index=109) -> (element=w1142:u8)
      n515 = Index Array(array=w1131, index=108) -> (element=w1143:u8)
      n516 = call "Process Data In 2 Byte Chunks.vi"("DATA IN"=w1130) -> ("Data Out"=w1128:u16[])  [unwired: 10 in]
      n517 = Join Numbers(hi=w1142, lo=w1143) -> ((hi.lo)=w1141:u16)
      n518 = Index Array(array=w1128) -> (element #1=w1127:u16, element #2=w1126:u16, element #3=w1125:u16, element #4=w1124:u16, element #5=w1123:u16, element #6=w1122:u16, element #7=w1121:u16, element #8=w1120:u16, element #9=w1119:u16, element #10=w1118:u16, element #11=w1117:u16, element #12=w1116:u16)  [unwired: 12 in]
      n519 = for {
        N: 15 -> [_]
        shift-right: [w1214] -> w1158
        shift-left: "" -> [w1215]
        tunnel: w1160 -> [w1212]
        i -> [w1211]
        w1205 = 2 ("index")
        n520 = Multiply(x=w1211, y=w1205) -> (x*y=w1204:i32)
        n521 = Array Subset(array=w1212, index=w1204, length=w1205) -> (w1210:u8[])
        n522 = Array To Cluster(array=w1210) -> (cluster=w1208:cluster{"[0]":u8, "[1]":u8})
        n523 = Unbundle By Name(w1208) -> ("[1]"=w1206:u8, "[0]"=w1207:u8)
        n524 = Join Numbers(hi=w1206, lo=w1207) -> ((hi.lo)=w1209:u16)
        n525 = Format Into String(format string="Reserved[%02d]=0x%02x\r\n", initial string=w1215, w1211, w1209) -> (resulting string=w1214:string)  [unwired: 1 in, 1 out]
      }
      n526 = for {
        N: 15 -> [_]
        shift-right: [w1202] -> w1154
        shift-left: "" -> [w1203]
        tunnel: w1155 -> [w1200]
        i -> [w1199]
        w1193 = 2 ("index")
        n527 = Multiply(x=w1199, y=w1193) -> (x*y=w1192:i32)
        n528 = Array Subset(array=w1200, index=w1192, length=w1193) -> (w1198:u8[])
        n529 = Array To Cluster(array=w1198) -> (cluster=w1196:cluster{"[0]":u8, "[1]":u8})
        n530 = Unbundle By Name(w1196) -> ("[1]"=w1194:u8, "[0]"=w1195:u8)
        n531 = Join Numbers(hi=w1194, lo=w1195) -> ((hi.lo)=w1197:u16)
        n532 = Format Into String(format string="Reserved[%02d]=0x%02x\r\n", initial string=w1203, w1199, w1197) -> (resulting string=w1202:string)  [unwired: 1 in, 1 out]
      }
      n533 = for {
        N: 6 -> [_]
        shift-right: [w1190] -> w1147
        shift-left: "" -> [w1191]
        tunnel: w1152 -> [w1188]
        i -> [w1186]
        w1178 = 2 ("index")
        n534 = Multiply(x=w1186, y=w1178) -> (x*y=w1187:i32)
        n535 = Add(x=w1187, y=4) -> (x+y=w1185:i32)
        n536 = Array Subset(array=w1188, index=w1185, length=w1178) -> (w1184:u8[])
        n537 = Array To Cluster(array=w1184) -> (cluster=w1181:cluster{"[0]":u8, "[1]":u8})
        n538 = Unbundle By Name(w1181) -> ("[1]"=w1179:u8, "[0]"=w1180:u8)
        n539 = Join Numbers(hi=w1179, lo=w1180) -> ((hi.lo)=w1182:u16)
        n540 = Format Into String(format string="batteryStateCalStimOff[%02d]=0x%02x\r\n", initial string=w1191, w1186, w1182) -> (resulting string=w1190:string)  [unwired: 1 in, 1 out]
      }
      n541 = for {
        N: 6 -> [_]
        shift-right: [w1176] -> w1146
        shift-left: "" -> [w1177]
        tunnel: w1150 -> [w1174]
        i -> [w1172]
        w1164 = 2 ("index")
        n542 = Multiply(x=w1172, y=w1164) -> (x*y=w1173:i32)
        n543 = Add(x=w1173, y=4) -> (x+y=w1171:i32)
        n544 = Array Subset(array=w1174, index=w1171, length=w1164) -> (w1170:u8[])
        n545 = Array To Cluster(array=w1170) -> (cluster=w1167:cluster{"[0]":u8, "[1]":u8})
        n546 = Unbundle By Name(w1167) -> ("[1]"=w1165:u8, "[0]"=w1166:u8)
        n547 = Join Numbers(hi=w1165, lo=w1166) -> ((hi.lo)=w1168:u16)
        n548 = Format Into String(format string="batteryStateCalStimOn[%02d]=0x%02x\r\n", initial string=w1177, w1172, w1168) -> (resulting string=w1176:string)  [unwired: 1 in, 1 out]
      }
      n549 = Format Into String(format string="%stempMinThreshold=0x%02x\r\ntempWarningThresholdl=0x%02x\r\ntempCriticalThresholdl=0x%02x\r\ntempAbortThresholdl=0x%02x\r\nthermOffsetMinimum=0x%02x\r\nthermOffsetMaximum=0x%02x\r\nthermBiasMinimum=0x%02x\r\nthermBiasMaximum=0x%02x\r\nthermInputMinimum=0x%02x\r\nthermInputMaximum=0x%02x\r\nbatteryIncreasePreCharge=0x%02x\r\nbatteryIncreaseConstandCurrent=0x%02x\r\n%s%s%svrectMeasurementCal=0x%02x\r\n", w1158, w1127, w1126, w1125, w1124, w1123, w1122, w1121, w1120, w1119, w1118, w1117, w1116, w1154, w1147, w1146, w1141) -> (resulting string=w1162:string)  [unwired: 2 in, 1 out]
    }
    frame 59 {
      # "SET_GENERAL_CALIBRATION"
    }
    frame 60 {
      # "GET_TRIM_LIST"
      n550 = Array To Cluster(array=w1219) -> (cluster=w1224:T6)
      n551 = Unbundle By Name(w1224) -> ("DATA[0]"=w1222:u8, "DATA[1]"=w1221:u8)
      n552 = case shown="0, Default" w1222 {
        tunnel: w1219 -> [w1229 w1254]
        tunnel: [w1227 w1252] -> w1223
        tunnel: w1221 -> [w1226 _]
        frame 0, Default {
          n553 = for {
            N: w1226 -> [_]
            shift-right: [w1243] -> w1227
            shift-left: "" -> [w1244]
            tunnel: w1229 -> [w1241]
            i -> [w1239]
            w1232 = 3 ("index")
            n554 = Multiply(x=w1239, y=w1232) -> (x*y=w1240:i32)
            n555 = Add(x=w1240, y=2) -> (x+y=w1238:i32)
            n556 = Array Subset(array=w1241, index=w1238, length=w1232) -> (w1237:u8[])
            n557 = Array To Cluster(array=w1237) -> (cluster=w1235:cluster{"[0]":u8, "[1]":u8, "[2]":u8})
            n558 = Unbundle By Name(w1235) -> ("[1]"=w1233:u8, "[0]"=w1234:u8, "[2]"=w1230:u8)
            n559 = Join Numbers(hi=w1233, lo=w1234) -> ((hi.lo)=w1231:u16)
            n560 = Format Into String(format string="Address=0x%04x\r\nData=0x%02x\r\n", initial string=w1244, w1231, w1230) -> (resulting string=w1243:string)  [unwired: 1 in, 1 out]
          }
        }
        frame 2 {
          n561 = Array To Cluster(array=w1254) -> (cluster=w1255:T12)
          n562 = Unbundle By Name(w1255) -> ("DATA[2]"=w1253:u8, "DATA[3]"=w1251:u8, "DATA[4]"=w1250:u8, "DATA[5]"=w1249:u8, "DATA[6]"=w1248:u8, "DATA[7]"=w1247:u8, "DATA[8]"=w1246:u8)
          n563 = Join Numbers(hi=w1247, lo=w1246) -> ((hi.lo)=w1245:u16)
          n564 = Format Into String(format string="BG_TRIM=0x%02x\r\nPGO_TRIM=0x%02x\r\nCASN_TRIM=0x%02x\r\nCASP_TRIM=0x%02x\r\nHVDDL_TRIM=0x%02x\r\nGLOBAL_GAIN_TRIM=0x%04x\r\n", w1253, w1251, w1250, w1249, w1248, w1245) -> (resulting string=w1252:string)  [unwired: 2 in, 1 out]
        }
      }
      n565 = Format Into String(format string="ListNum=%d\r\nListLen=%d\r\n%s", w1222, w1221, w1223) -> (resulting string=w1220:string)  [unwired: 2 in, 1 out]
    }
    frame 61 {
      # "SET_TRIM_LIST"
    }
    frame 62 {
      # "GET_COUNTER"
      n566 = Array To Cluster(array=w1269) -> (cluster=w1268:T4)
      n567 = Unbundle By Name(w1268) -> ("DATA[0]"=w1267:u8, "DATA[2]"=w1265:u8, "DATA[3]"=w1266:u8, "DATA[4]"=w1263:u8, "DATA[5]"=w1264:u8)
      n568 = Join Numbers(hi=w1264, lo=w1263) -> ((hi.lo)=w1262:u16)
      n569 = Join Numbers(hi=w1266, lo=w1265) -> ((hi.lo)=w1261:u16)
      n570 = Join Numbers(hi=w1262, lo=w1261) -> ((hi.lo)=w1260:u32)
      n571 = Format Into String(format string="eventCounterID=%d\r\neventCount=%d\r\n", w1267, w1260) -> (resulting string=w1270:string)  [unwired: 2 in, 1 out]
    }
    frame 63 {
      # "SET_COUNTER"
    }
    frame 64 {
      # "GET_TEST_STIMULATION"
      n572 = Index Array(array=w1276, index #1=0 ("index")) -> (element #1=w1279:u8, element #2=w1278:u8, element #3=w1277:u8)  [unwired: 2 in]
      n573 = for {
        N: 4 -> [_]
        shift-right: [w1316] -> w1275
        shift-left: "" -> [w1317]
        tunnel: w1276 -> [w1306]
        i -> [w1307]
        w1286 = 8 ("index")
        w1321 = 35 ("length")
        n574 = Multiply(x=w1307, y=w1321) -> (x*y=w1319:i32)
        n575 = Add(x=3 ("index"), y=w1319) -> (x+y=w1320:i32)
        n576 = Array Subset(array=w1306, index=w1320, length=w1321) -> (w1304:u8[])
        n577 = Array To Cluster(array=w1304) -> (cluster=w1299:T13)
        n578 = Array Subset(array=w1304, index=5, length=26) -> (w1310:u8[])
        n579 = Unbundle By Name(w1299) -> ("[31]"=w1298:u8, "[32]"=w1297:u8, "[33]"=w1296:u8, "[34]"=w1293:u8, "[35]"=w1292:u8, "[36]"=w1288:u8, "[37]"=w1287:u8)
        n580 = Unbundle By Name(w1299) -> ("[3]"=w1302:u8, "[4]"=w1303:u8)
        n581 = To Unsigned Word Integer(number=w1303) -> (unsigned 16bit integer=w1315:u16)
        n582 = for {
          N: 26 -> [_]
          tunnel: w1310 -> [w1322] mode=indexing
          shift-right: [w1328] -> w1300
          shift-left: "" -> [w1329]
          tunnel: w1307 -> [w1323]
          i -> [w1326]
          n583 = case shown="3" w1323 {
            tunnel: ["ChannelPercentagePA[CH%02d]=%d\\r\\n" ("format string") "ChannelPercentagePB[CH%02d]=%d\\r\\n" ("format string") "ChannelPercentagePC[CH%02d]=%d\\r\\n" ("format string") "ChannelPercentagePD[CH%02d]=%d\\r\\n" ("format string")] -> w1327
            frame 0, Default {
            }
            frame 1 {
            }
            frame 2 {
            }
            frame 3 {
            }
          }
          n584 = To Byte Integer(number=w1322) -> (8bit integer=w1324:i8)
          n585 = Increment(x=w1326) -> (x+1=w1325:i32)
          n586 = Format Into String(format string=w1327, initial string=w1329, w1325, w1324) -> (resulting string=w1328:string)  [unwired: 1 in, 1 out]
        }
        n587 = To Unsigned Word Integer(number=w1292) -> (unsigned 16bit integer=w1294:u16)
        n588 = To Unsigned Word Integer(number=w1287) -> (unsigned 16bit integer=w1290:u16)
        n589 = Logical Shift(y=8 ("index"), x=w1315) -> (x << y=w1314:u16)
        n590 = Logical Shift(y=w1286, x=w1294) -> (x << y=w1295:u16)
        n591 = Logical Shift(y=w1286, x=w1290) -> (x << y=w1289:u16)
        n592 = Add(x=w1302, y=w1314) -> (x+y=w1301:u16)
        n593 = Add(x=w1293, y=w1295) -> (x+y=w1291:u16)
        n594 = Add(x=w1288, y=w1289) -> (x+y=w1285:u16)
        n595 = Format Into String(format string="\r\n-- PULSE PB --\r\nAmplitude=%d\r\n%s\r\nStimWidth=%d\r\nInterphaseDelay=%d\r\nRecoveryRatioSelect=%d\r\nPassiveRecoveryWidth=%d\r\nCBCWidth=%d", initial string=w1317, w1301, w1300, w1298, w1297, w1296, w1291, w1285) -> (resulting string=w1316:string)  [unwired: 1 in, 1 out]
      }
      n596 = Format Into String(format string="FrequencyIndex=%d\r\nComplianceVoltage=%d\r\nNumPulses=%d\r\n%s", w1279, w1278, w1277, w1275) -> (resulting string=w1284:string)  [unwired: 2 in, 1 out]
    }
    frame 65 {
      # "SET_TEST_STIMULATION"
    }
    frame 66 {
      # "GET_TITRATION_STIMULATION"
      n597 = Index Array(array=w1338, index #1=0 ("index")) -> (element #1=w1342:u8, element #2=w1341:u8)  [unwired: 1 in]
      n598 = for {
        N: 4 -> [_]
        shift-right: [w1368] -> w1337
        shift-left: "" -> [w1369]
        tunnel: w1338 -> [w1359]
        i -> [w1360]
        w1348 = 8 ("index")
        w1373 = 30 ("length")
        n599 = Multiply(x=w1360, y=w1373) -> (x*y=w1371:i32)
        n600 = Add(x=2 ("index"), y=w1371) -> (x+y=w1372:i32)
        n601 = Array Subset(array=w1359, index=w1372, length=w1373) -> (w1357:u8[])
        n602 = Array To Cluster(array=w1357) -> (cluster=w1353:T14)
        n603 = Array Subset(array=w1357, index=6, length=26) -> (w1363:u8[])
        n604 = Unbundle By Name(w1353) -> ("[2]"=w1355:u8, "[3]"=w1356:u8, "[4]"=w1350:u8, "[5]"=w1349:u8)
        n605 = To Unsigned Word Integer(number=w1356) -> (unsigned 16bit integer=w1367:u16)
        n606 = To Unsigned Word Integer(number=w1349) -> (unsigned 16bit integer=w1351:u16)
        n607 = for {
          N: 26 -> [_]
          tunnel: w1363 -> [w1374] mode=indexing
          shift-right: [w1380] -> w1346
          shift-left: "" -> [w1381]
          tunnel: w1360 -> [w1375]
          i -> [w1378]
          n608 = case shown="3" w1375 {
            tunnel: ["channelPercentagePA[CH%02d]=%d\\r\\n" ("format string") "channelPercentagePB[CH%02d]=%d\\r\\n" ("format string") "channelPercentagePC[CH%02d]=%d\\r\\n" ("format string") "channelPercentagePD[CH%02d]=%d\\r\\n" ("format string")] -> w1379
            frame 0, Default {
            }
            frame 1 {
            }
            frame 2 {
            }
            frame 3 {
            }
          }
          n609 = To Byte Integer(number=w1374) -> (8bit integer=w1376:i8)
          n610 = Increment(x=w1378) -> (x+1=w1377:i32)
          n611 = Format Into String(format string=w1379, initial string=w1381, w1377, w1376) -> (resulting string=w1380:string)  [unwired: 1 in, 1 out]
        }
        n612 = Logical Shift(y=w1348, x=w1367) -> (x << y=w1366:u16)
        n613 = Logical Shift(y=w1348, x=w1351) -> (x << y=w1352:u16)
        n614 = Add(x=w1355, y=w1366) -> (x+y=w1354:u16)
        n615 = Add(x=w1350, y=w1352) -> (x+y=w1347:u16)
        n616 = Format Into String(format string="\r\n-- TITR_PULSE PB --\r\nAmplitude=%d\r\npulseWidth=%d\r\n%s", initial string=w1369, w1354, w1347, w1346) -> (resulting string=w1368:string)  [unwired: 1 in, 1 out]
      }
      n617 = Format Into String(format string="frequencyIndex=%d\r\nnumPulses=%d\r\n%s", w1342, w1341, w1337) -> (resulting string=w1345:string)  [unwired: 2 in, 1 out]
    }
    frame 67 {
      # "SET_TITRATION_STIMULATION"
    }
    frame 68 {
      # "GET_RAMP_TIME"
      n618 = Array To Cluster(array=w1396) -> (cluster=w1395:cluster{"DATA[0]":u8, "DATA[1]":u8})
      n619 = Unbundle By Name(w1395) -> ("DATA[0]"=w1392:u8, "DATA[1]"=w1391:u8)
      n620 = To Unsigned Word Integer(number=w1391) -> (unsigned 16bit integer=w1390:u16)
      n621 = Logical Shift(y=8 ("index"), x=w1390) -> (x << y=w1394:u16)
      n622 = Add(x=w1392, y=w1394) -> (x+y=w1389:u16)
      n623 = Format Into String(format string="RampTime=%d\r\n", w1389) -> (resulting string=w1397:string)  [unwired: 2 in, 1 out]
    }
    frame 69 {
      # "SET_RAMP_TIME"
    }
    frame 70 {
      # "GET_VBAT"
      n624 = Array To Cluster(array=w1403) -> (cluster=w1409:cluster{"DATA[0]":u8, "DATA[1]":u8})
      n625 = Unbundle By Name(w1409) -> ("DATA[0]"=w1406:u8, "DATA[1]"=w1405:u8)
      n626 = To Unsigned Word Integer(number=w1405) -> (unsigned 16bit integer=w1404:u16)
      n627 = Logical Shift(y=8 ("index"), x=w1404) -> (x << y=w1408:u16)
      n628 = Add(x=w1406, y=w1408) -> (x+y=w1402:u16)
      n629 = Format Into String(format string="vbat=%d\r\n", w1402) -> (resulting string=w1411:string)  [unwired: 2 in, 1 out]
    }
    frame 71 {
      (unwired) "" ("format string")
      # "Not yet documented"
      # "SET_SOFTWARE_DESCRIPTION_BLOCK"
    }
    frame 72 {
      (unwired) "FrequencyIndex=%s\r\n" ("format string")
      # "Not yet documented"
      # "GET_SOFTWARE_DESCRIPTION_BLOCK"
    }
    frame 73 {
      # "WRITE_MEMORY"
    }
    frame 74 {
      # "READ_MEMORY"
      n630 = Array To Cluster(array=w1424) -> (cluster=w1440:T15)
      n631 = Unbundle By Name(w1440) -> ("DATA[3]"=w1437:u8, "DATA[2]"=w1436:u8, "DATA[1]"=w1435:u8, "DATA[0]"=w1434:u8, "DATA[4]"=w1426:u8, "DATA[5]"=w1427:u8)
      n632 = Array Subset(array=w1424, index=6, length=64 ("index")) -> (w1416:u8[])
      n633 = Join Numbers(hi=w1437, lo=w1436) -> ((hi.lo)=w1439:u16)
      n634 = Join Numbers(hi=w1435, lo=w1434) -> ((hi.lo)=w1438:u16)
      n635 = Byte Array To String(unsigned byte array=w1416) -> (string=w1419:string)
      n636 = To Unsigned Word Integer(number=w1427) -> (unsigned 16bit integer=w1428:u16)
      n637 = Index Array(array=w1416, index #1=0 ("index"), index #2=1 ("index")) -> (element #1=w1420:u8, element #2=w1417:u8)
      n638 = Join Numbers(hi=w1439, lo=w1438) -> ((hi.lo)=w1431:u32)
      n639 = Logical Shift(y=8 ("index"), x=w1428) -> (x << y=w1430:u16)
      n640 = Add(x=w1426, y=w1430) -> (x+y=w1425:u16)
      n641 = Format Into String(format string="address=%d\r\nlength=%d\r\ndata0=%d\r\ndata1=%d\r\n%s", w1431, w1425, w1420, w1417, w1419) -> (resulting string=w1432:string)  [unwired: 2 in, 1 out]
    }
    frame 75 {
      (unwired) "" ("format string")
      # "Not yet documented"
      # "RESET_xPG"
    }
    frame 76 {
      (unwired) "" ("format string")
      # "Not yet documented"
      # "ERASE_FLASH_BLOCK"
    }
    frame 77 {
      (unwired) "" ("format string")
      # "Not yet documented"
      # "WRITE_VECTORS"
    }
    frame 78 {
      (unwired) "" ("format string")
      # "Not yet documented"
      # "READ_VECTORS"
    }
    frame 79 {
      # "DIAGNOSTIC_DATA"
      n642 = Index Array(array=w1447, index=1) -> (element=w1449:u8)
      n643 = case shown="5, Default" w1449 {
        tunnel: [w1461 "Unsupported State" w1478 w1495] -> w1448
        tunnel: w1447 -> [w1458 _ w1477 w1487]
        frame 0, 1 {
          # "Capacitor Data, BG Impedance"
          n644 = Array Subset(array=w1458, index=2, length=53) -> (w1456:u8[])
          n645 = for {
            N: 26 -> [_]
            shift-right: [w1473] -> w1454
            shift-left: w1456 -> [w1475]
            shift-right: [w1462] -> w1451
            shift-left: "" -> [w1463]
            i -> [w1466]
            n646 = Split 1D Array(array=w1475, index=2) -> (first subarray=w1472:u8[], second subarray=w1473:u8[])
            n647 = Increment(x=w1466) -> (x+1=w1465:i32)
            n648 = Index Array(array=w1472, index #1=1 ("index"), index #2=0 ("index")) -> (element #1=w1468:u8, element #2=w1469:u8)
            n649 = Join Numbers(hi=w1468, lo=w1469) -> ((hi.lo)=w1464:u16)
            n650 = Format Into String(format string="Channel%d Voltage=%d\\r\\n", initial string=w1463, w1465, w1464) -> (resulting string=w1462:string)  [unwired: 1 in, 1 out]
          }
          n651 = Index Array(array=w1454) -> (element=w1452:u8)  [unwired: 1 in]
          n652 = Format Into String(format string="%sData Valid=%d", w1451, w1452) -> (resulting string=w1461:string)  [unwired: 2 in, 1 out]
        }
        frame 5, Default {
        }
        frame 2 {
          # "VBat Data"
          n653 = Array To Cluster(array=w1477) -> (cluster=w1480:T6)
          n654 = Unbundle By Name(w1480) -> ("DATA[3]"=w1481:u8, "DATA[2]"=w1482:u8)
          n655 = Join Numbers(hi=w1481, lo=w1482) -> ((hi.lo)=w1479:u16)
          n656 = Format Into String(format string="VoltageReading=%d\r\n", w1479) -> (resulting string=w1478:string)  [unwired: 2 in, 1 out]
        }
        frame 3 {
          # "Thermistor Data"
          n657 = Array To Cluster(array=w1487) -> (cluster=w1488:T6)
          n658 = Unbundle By Name(w1488) -> ("DATA[3]"=w1493:u8, "DATA[2]"=w1494:u8, "DATA[5]"=w1491:u8, "DATA[4]"=w1492:u8, "DATA[7]"=w1489:u8, "DATA[6]"=w1490:u8)
          n659 = Join Numbers(hi=w1493, lo=w1494) -> ((hi.lo)=w1486:u16)
          n660 = Join Numbers(hi=w1491, lo=w1492) -> ((hi.lo)=w1485:u16)
          n661 = Join Numbers(hi=w1489, lo=w1490) -> ((hi.lo)=w1484:u16)
          n662 = Format Into String(format string="ThermBias=%d\r\nThermInput=%d\r\nThermOffset=%d", w1486, w1485, w1484) -> (resulting string=w1495:string)  [unwired: 2 in, 1 out]
        }
      }
    }
    frame 80 {
      # "SET_BACKGROUND_IMPEDANCE"
    }
    frame 81 {
      # "GET_BACKGROUND_IMPEDANCE"
      n663 = Array To Cluster(array=w1505) -> (cluster=w1504:T16)
      n664 = Unbundle By Name(w1504) -> ("DATA[0]"=w1500:u8, "DATA[1]"=w1502:u8)
      n665 = Greater Than 0?(x=w1502) -> (x > 0?=w1503:bool)
      n666 = case shown="False" w1503 {
        tunnel: ["disabled" "enabled"] -> w1501
        frame False {
        }
        frame True {
        }
      }
      n667 = Format Into String(format string="bgiAmplitude=%d\r\nenabled=%s\r\n", w1500, w1501) -> (resulting string=w1507:string)  [unwired: 2 in, 1 out]
    }
    frame 32682 {
      # "Undefined"
    }
  }
  "CP_DATA" <- w2
  n668 = Unbundle By Name(w21) -> ("respToken"=w7:u8, "cmdToken"=w9:u16, "b1ChkSum"=w27:u8, "b1ChkSumCalc"=w26:u8, "tChkSum"=w25:u8, "tChkSumCalc"=w24:u8)
  n669 = call <vilib>:"Trim Whitespace.vi"("string"=w29) -> ("trimmed string"=→"Data":string)  [unwired: 1 in]
  n670 = Equal?(x=w27, y=w26) -> (x = y?=→"bChecksum Valid":bool)
  n671 = Equal?(x=w25, y=w24) -> (x = y?=→"tChecksum Valid":bool)
  n672 = call "MICS Response Lookup.vi"("Token"=w7) -> ("description"=w5:string, "name"=w6:string)  [unwired: 5 in, 3 out]
  n673 = call "MICS Command Lookup.vi"("token"=w9) -> ("command"=→"Response Token":string)  [unwired: 5 in, 4 out]
  n674 = Concatenate Strings(w6, "\n" ("string"), w5) -> (→"Response Code":string)
  "error out" <- "error in (no error)"
